vi "try_Select Enum Item.vi"() -> ()   [LabVIEW 2020]
panel:
  in  "Enum":T1(ring)
  # "Scenario\nWhen navigating an enum with a large number of items, it can be difficult to find the item you want.\n\nInstructions\n1. Right-click the enum and choose Select Item.\n2. In the UI that appears, type characters to filter the list.\n3. Select an item in the list by either double-clicking on it, or using the arrow keys and pressing Enter. The value of the enum will change to the one you selected."
  # "Close this VI when you are done with the demo."
  # "You do not need to save changes to this VI."
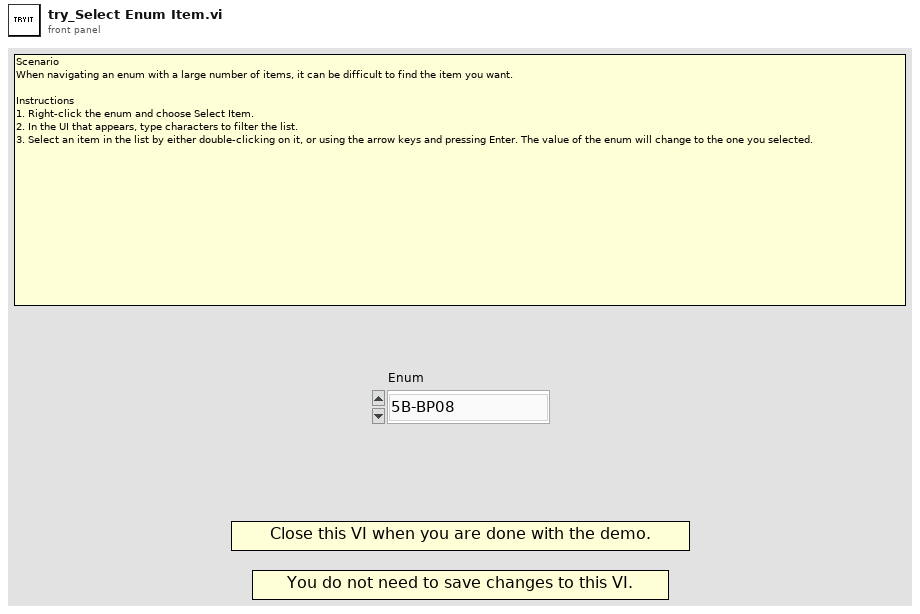
[diagram p1: front panel]
types:
  T1 = enum16{"5B-BP08", "5B-BP16", "5B30", "5B31", "5B32", "5B34", "5B37", "5B38", "5B39", "5B40", "5B41", "5B45", "5B46", "5B47", "5B49", "AMUX-64T", "AT-1120", "AT-1212", "AT-232/2", "AT-232/2 NSI", "AT-232/4", "AT-232/4 NSI", "AT-232I/2", "AT-232I/4", "AT-485/2", "AT-485/2 NSI", "AT-485/4", "AT-485/4 NSI", "AT-485I/2", "AT-485I/4", "AT-5102", "AT-5411", "AT-5431", "AT-6020/OEM1", "AT-6022E", "AT-AI-16XE-10", "AT-AO-10", "AT-AO-6", "AT-CAN", "AT-CAN/2", "AT-DIO-32F", "AT-DIO-32HS", "AT-DSP2200", "AT-GPIB", "AT-GPIB/TNT", "AT-GPIB/TNT (PnP)", "AT-GPIB/TNT+", "AT-MIO-16DE-10", "AT-MIO-16DH-25", "AT-MIO-16DH-9", "AT-MIO-16DL-25", "AT-MIO-16DL-9", "AT-MIO-16E-1", "AT-MIO-16E-10", "AT-MIO-16E-2", "AT-MIO-16F-5", "AT-MIO-16H-15", "AT-MIO-16H-25", "AT-MIO-16H-9", "AT-MIO-16L-15", "AT-MIO-16L-25", "AT-MIO-16L-9", "AT-MIO-16X", "AT-MIO-16XE-10", "AT-MIO-16XE-50", "AT-MIO-64E-3", "AT-MIO-64F-5", "AT-MXI", "AT-MXI-2", "BNC-2080", "BNC-2081", "BNC-2082", "BNC-2090", "BNC-2090A", "BNC-2095", "BNC-2096", "BNC-2110", "BNC-2111", "BNC-2115", "BNC-2120", "BNC-2121", "BNC-2140", "BNC-2142", "CAL-4353", "CB-100", "CB-27", "CB-27T", "CB-37F-HVD", "CB-50", "CB-50LC", "CB-50LP", "CB-68LP", "CB-68LPR", "CB-68T", "CEC USBDAQ/108", "CEC USBDAQ/109", "CF-6004", "CVS-1450", "CVS-1451RT", "CVS-1454", "CVS-1455", "CVS-1457RT", "CVS-1458RT", "CVS-1459RT", "CompactRIO PROFINET Slave Module", "DAQCard-1200", "DAQCard-4050", "DAQCard-4350", "DAQCard-4502", "DAQCard-500", "DAQCard-5102", "DAQCard-516", "DAQCard-5402", "DAQCard-6023E", "DAQCard-6024E", "DAQCard-6034E", "DAQCard-6035E", "DAQCard-6036E", "DAQCard-6062E", "DAQCard-6533", "DAQCard-6601", "DAQCard-6715", "DAQCard-6830", "DAQCard-700", "DAQCard-AI-16E-4", "DAQCard-AI-16XE-50", "DAQCard-AO-2DC", "DAQCard-DIO-24", "DAQPad-1200", "DAQPad-4350 for USB", "DAQPad-4351 for IEEE 1394", "DAQPad-4352 for USB", "DAQPad-5102", "DAQPad-5112 for IEEE 1394", "DAQPad-6015 for USB", "DAQPad-6015 for USB w/BNC Term", "DAQPad-6015 for USB w/Mass Term", "DAQPad-6015 for USB w/Screw Term", "DAQPad-6016 for USB w/Screw Term", "DAQPad-6020E for USB w/BNC Term", "DAQPad-6020E for USB w/Mass Term", "DAQPad-6024E for USB w/BNC Term", "DAQPad-6024E for USB w/Mass Term", "DAQPad-6025E for USB w/BNC Term", "DAQPad-6025E for USB w/Mass Term", "DAQPad-6036E for USB w/BNC Term", "DAQPad-6036E for USB w/Mass Term", "DAQPad-6052E for Ethernet w/BNC Term", "DAQPad-6052E for Ethernet w/Mass Term", "DAQPad-6052E for IEEE 1394 w/BNC Term", "DAQPad-6052E for IEEE 1394 w/Mass Term", "DAQPad-6052E for USB w/BNC Term", "DAQPad-6052E for USB w/Mass Term", "DAQPad-6070E for IEEE 1394 w/BNC Term", "DAQPad-6070E for IEEE 1394 w/Mass Term", "DAQPad-6507 for USB", "DAQPad-6508 for USB", "DAQPad-6533 for IEEE 1394", "DAQPad-6713 for IEEE 1394 w/Mass Term", "DAQPad-MIO-16XE-50", "DAQPad-TB-52", "EISA-A2000", "EISA-GPIB", "ENET-232/2", "ENET-232/4", "ENET-485/2", "ENET-485/4", "ENET-7344", "ENET-9205", "ENET-9205 DSUB", "ENET-9206", "ENET-9211", "ENET-9213", "ENET-9215", "ENET-9215 BNC", "ENET-9219", "ENET-9234", "ENET-9237", "ENET-9421", "ENET-9421 DSUB", "ENET-9472", "ENET-9472 DSUB", "ENET-9481", "ER-16", "ER-8", "FP-1000", "FP-1001", "FP-1300", "FP-1600", "FP-1601", "FP-2000", "FP-2010", "FP-2015", "FP-3000", "FP-AI-100", "FP-AI-102", "FP-AI-110", "FP-AI-111", "FP-AI-112", "FP-AIO-600", "FP-AIO-610", "FP-AO-200", "FP-AO-210", "FP-CTR-500", "FP-CTR-502", "FP-DI-300", "FP-DI-301", "FP-DI-330", "FP-DIO-550", "FP-DO-400", "FP-DO-401", "FP-DO-403", "FP-DO-410", "FP-PG-522", "FP-PWM-520", "FP-QUAD-510", "FP-RLY-420", "FP-RLY-422", "FP-RTD-122", "FP-RTD-124", "FP-SG-140", "FP-TB-1 for USB", "FP-TC-120", "FP-TC-125", "FW-7344", "GPIB-1394", "GPIB-ENET/100", "GPIB-PCII", "GPIB-PCII/IIA", "GPIB-USB", "GPIB-USB-A", "GPIB-USB-B", "GPIB-USB-HS", "GPIB-VXI/C", "IC-3120", "IC-3121", "IC-3171", "IC-3172", "IC-3173", "ISC-1780", "ISC-1780 (Color)", "ISC-1781", "ISC-1781 (Color)", "ISC-1782", "ISC-1782 (Color)", "ISC-1783", "ISC-1783 (Color)", "Lab-PC", "Lab-PC+", "Lab-PC-1200", "Lab-PC-1200AI", "MC-DIO-24", "MC-DIO-32F", "MC-MIO-16H-15", "MC-MIO-16H-25", "MC-MIO-16L-15", "MC-MIO-16L-25", "MC-MIO-16L-9", "MCC USB-488", "NB-MIO-16H-9", "NEC-AI-16E-4", "NEC-AI-16XE-50", "NEC-GPIB/TNT", "NEC-GPIB/TNT (PnP)", "NEC-MIO-16E-4", "NEC-MIO-16XE-50", "NET2280", "NI 1483", "NI 1485", "NI 1712", "NI 1722", "NI 1732", "NI 1742", "NI 1744", "NI 1752", "NI 1754", "NI 1762", "NI 1764", "NI 1772", "NI 1772C", "NI 1774", "NI 1774C", "NI 1776", "NI 1776C", "NI 1778", "NI 17XX Series Smart Camera", "NI 2810", "NI 2811", "NI 2812", "NI 2813", "NI 2814", "NI 2815", "NI 2816", "NI 2817", "NI 2833", "NI 2834", "NI 2865", "NI 4472 for IEEE 1394", "NI 5731", "NI 5732", "NI 5733", "NI 5734", "NI 5741", "NI 5742", "NI 5751", "NI 5751B", "NI 5752", "NI 5752B", "NI 5753", "NI 5753 (-01) AC", "NI 5753 (-02) DC", "NI 5761", "NI 5771", "NI 5772", "NI 5781", "NI 5782", "NI 5782 (DC)", "NI 5783", "NI 5791", "NI 5792", "NI 5793", "NI 6224 for Ethernet w/BNC Term", "NI 6224 for Ethernet w/Mass Term", "NI 6224 for Ethernet w/SCXI Term", "NI 6225 for Ethernet", "NI 6226 for Ethernet", "NI 6581", "NI 6581B", "NI 6583", "NI 6584", "NI 6585", "NI 6585B", "NI 6587", "NI 6588", "NI 6589", "NI 7451", "NI 9145", "NI 9146", "NI 9147", "NI 9148", "NI 9149", "NI 9154", "NI 9155", "NI 9157", "NI 9159", "NI 9201", "NI 9201 D-Sub", "NI 9201 cRIO", "NI 9203", "NI 9203 cRIO", "NI 9205", "NI 9205 (DSUB)", "NI 9205 D-Sub", "NI 9205 cRIO", "NI 9206", "NI 9206 cRIO", "NI 9207", "NI 9208", "NI 9209", "NI 9210", "NI 9211", "NI 9211 cRIO", "NI 9212", "NI 9213", "NI 9214", "NI 9215", "NI 9215 (BNC)", "NI 9215 BNC", "NI 9215 cRIO", "NI 9215E", "NI 9216", "NI 9217", "NI 9217 cRIO", "NI 9218", "NI 9219", "NI 9219 LEMO", "NI 9219 cRIO", "NI 9219E", "NI 9220", "NI 9220 cDAQ", "NI 9221", "NI 9221 (DSUB)", "NI 9221 (DSUB) cRIO", "NI 9221 cRIO", "NI 9222", "NI 9223", "NI 9223 cDAQ", "NI 9224", "NI 9225", "NI 9225 cRIO", "NI 9226", "NI 9227", "NI 9228", "NI 9229", "NI 9229 (BNC)", "NI 9229 BNC", "NI 9229 cRIO", "NI 9230", "NI 9230 BNC cDAQ", "NI 9232", "NI 9232 BNC cDAQ", "NI 9232 cDAQ", "NI 9232E", "NI 9233", "NI 9234", "NI 9234B", "NI 9234E", "NI 9235", "NI 9236", "NI 9237", "NI 9237 cRIO", "NI 9237 with D-Sub", "NI 9238", "NI 9239", "NI 9239 (BNC)", "NI 9239 BNC", "NI 9239 cRIO", "NI 9242", "NI 9244", "NI 9246", "NI 9247", "NI 9250", "NI 9251", "NI 9251 Mini XLR cDAQ", "NI 9260", "NI 9263", "NI 9263 (BNC)", "NI 9263 cRIO", "NI 9264", "NI 9264 D-sub", "NI 9264 cRIO", "NI 9265", "NI 9265 cRIO", "NI 9265E", "NI 9266", "NI 9269", "NI 9344", "NI 9361", "NI 9375", "NI 9375 (DSUB)", "NI 9381 DSUB", "NI 9401", "NI 9401 cRIO", "NI 9402", "NI 9402 cRIO", "NI 9403", "NI 9403 cRIO", "NI 9411", "NI 9411 cRIO", "NI 9421", "NI 9421 (DSUB)", "NI 9421 D-Sub", "NI 9421 cRIO", "NI 9422", "NI 9422 cRIO", "NI 9423", "NI 9423 cRIO", "NI 9425", "NI 9425 cRIO", "NI 9426", "NI 9426 cRIO", "NI 9435", "NI 9435 cRIO", "NI 9436", "NI 9437", "NI 9467", "NI 9469", "NI 9472", "NI 9472 (DSUB)", "NI 9472 D-Sub", "NI 9472 cRIO", "NI 9474", "NI 9474 cRIO", "NI 9475", "NI 9476", "NI 9476 cRIO", "NI 9477", "NI 9477 cRIO", "NI 9478 cRIO", "NI 9481", "NI 9481 cRIO", "NI 9481E", "NI 9482", "NI 9485", "NI 9485 cRIO", "NI 9501", "NI 9502", "NI 9503", "NI 9505", "NI 9512", "NI 9514", "NI 9516", "NI 9770", "NI 9775", "NI 9792", "NI 9795", "NI 9802 cRIO", "NI 9841", "NI 9853", "NI 9860", "NI 9861", "NI 9862", "NI 9866", "NI 9870 cRIO", "NI 9870E", "NI 9871 cRIO", "NI 9871E", "NI Bluetooth Toolkit", "NI CAN Interfaces (Series 2)", "NI CVS-1450 Series", "NI DeviceNet Interfaces", "NI ELVIS II", "NI ELVIS II+", "NI EVS-1460 Series", "NI ExpressCard-8360", "NI ExpressCard-8420/2", "NI ExpressCard-8421/2", "NI ExpressCard-GPIB", "NI PCI-8511 CAN/LS1", "NI PCI-8511 CAN/LS2", "NI PCI-8512 CAN/HS1", "NI PCI-8512 CAN/HS2", "NI PCI-8513 CAN/XS1", "NI PCI-8513 CAN/XS2", "NI PCI-8516 LIN/2", "NI PCI-8517 FlexRay2", "NI PCIe-1427", "NI PCIe-1429", "NI PCIe-1430", "NI PCIe-1433", "NI PCIe-4065", "NI PCIe-5122", "NI PCIe-5142", "NI PCIe-6250", "NI PCIe-6251", "NI PCIe-6259", "NI PCIe-6344R", "NI PCIe-6346R", "NI PCIe-6509", "NI PCIe-6535", "NI PCIe-6536", "NI PCIe-6537", "NI PCIe-6542", "NI PCIe-6552", "NI PCIe-8231", "NI PCIe-8235", "NI PCIe-8253", "NI PCIe-8255R", "NI PCIe-GPIB", "NI PXI-4110", "NI PXI-4130", "NI PXI-4131A", "NI PXI-4132", "NI PXI-8511 CAN/LS1", "NI PXI-8511 CAN/LS2", "NI PXI-8512 CAN/HS1", "NI PXI-8512 CAN/HS2", "NI PXI-8513 CAN/XS1", "NI PXI-8513 CAN/XS2", "NI PXI-8516 LIN/2", "NI PXI-8517 FlexRay2", "NI PXIe-1062Q", "NI PXIe-1065", "NI PXIe-1436", "NI PXIe-1491", "NI PXIe-4112", "NI PXIe-4113", "NI PXIe-4136", "NI PXIe-4137", "NI PXIe-4138", "NI PXIe-4139", "NI PXIe-4140", "NI PXIe-4141", "NI PXIe-4142", "NI PXIe-4143", "NI PXIe-4144", "NI PXIe-4145", "NI PXIe-4154", "NI PXIe-4496", "NI PXIe-4498", "NI PXIe-5122", "NI PXIe-5142", "NI PXIe-5421", "NI PXIe-5422", "NI PXIe-5442", "NI PXIe-5450", "NI PXIe-5451", "NI PXIe-5452", "NI PXIe-5453", "NI PXIe-5455", "NI PXIe-5602", "NI PXIe-5612", "NI PXIe-5622", "NI PXIe-6251", "NI PXIe-6259", "NI PXIe-6535", "NI PXIe-6536", "NI PXIe-6537", "NI PXIe-6542", "NI PXIe-6552", "NI PXIe-8103", "NI PXIe-8105", "NI PXIe-8106", "NI PXIe-8130", "NI PXIe-8131", "NI PXIe-8234", "NI SoftMotion Controller for CANopen", "NI SoftMotion Controller for IEEE 1394", "NI TBX-2808", "NI USB 7845R", "NI USB 7845R OEM", "NI USB 7846R OEM", "NI USB-6341", "NI USB-6341 OEM", "NI USB-6343", "NI USB-6343 OEM", "NI USB-6351", "NI USB-6353", "NI USB-6356 (32 MS) (Screw Terminal)", "NI USB-6356 (32MS)", "NI USB-6356 (32MS) OEM", "NI USB-6356 (64 MS) (Screw Terminal)", "NI USB-6356 (64MS)", "NI USB-6361", "NI USB-6361 OEM", "NI USB-6363", "NI USB-6363 OEM", "NI USB-6366 (32 MS) (Screw Terminal)", "NI USB-6366 (32MS)", "NI USB-6366 (64 MS) (Screw Terminal)", "NI USB-6366 (64MS)", "NI USB-6366 (64MS) OEM", "NI USB-7846R", "NI USB-7855R", "NI USB-7855R OEM", "NI USB-7856R", "NI USB-7856R OEM", "NI USB-TC01", "NI USRP-2944R", "NI USRP-2954R", "NI WSN-3202", "NI WSN-3202 (programmable)", "NI WSN-3212", "NI WSN-3212 (programmable)", "NI WSN-3214", "NI WSN-3214 LV", "NI WSN-3226", "NI WSN-3226 (programmable)", "NI WSN-3230", "NI WSN-3231", "NI WSN-3234", "NI WSN-3234 LV", "NI WSN-9791", "NI WSN-9792 OEM", "NI myDAQ", "NI myDAQ Hardware", "NI myRIO", "NI roboRIO", "NI-1702", "NI-7931", "NI-7932", "NI-7935", "NI-9852", "NI-IMAQ for IEEE 1394 Cameras", "OEM USB-7931R", "OEM USB-7932R", "OEM USB-7933R", "PC-4350", "PC-516", "PC-AO-2DC", "PC-DIO-24", "PC-DIO-96", "PC-DIO-96PnP", "PC-FlexMotion-6C", "PC-LPM-16", "PC-LPM-16PnP", "PC-OPDIO-16", "PC-Servo-1P", "PC-Servo-2A", "PC-Servo-4A", "PC-Step-2CX", "PC-Step-2OX", "PC-Step-4CX", "PC-Step-4OX", "PC-TIO-10", "PCI-1200", "PCI-1405", "PCI-1407", "PCI-1408", "PCI-1409", "PCI-1410", "PCI-1411", "PCI-1412", "PCI-1413", "PCI-1422", "PCI-1423", "PCI-1424", "PCI-1426", "PCI-1428", "PCI-1588", "PCI-232/16", "PCI-232/2", "PCI-232/4", "PCI-232/8", "PCI-232I/2", "PCI-232I/4", "PCI-4021", "PCI-4060", "PCI-4065", "PCI-4070", "PCI-4351", "PCI-4451", "PCI-4452", "PCI-4453", "PCI-4454", "PCI-4461", "PCI-4462", "PCI-4472", "PCI-4472B", "PCI-4474", "PCI-4551", "PCI-4552", "PCI-485/2", "PCI-485/4", "PCI-485/8", "PCI-485I/2", "PCI-485I/4", "PCI-488", "PCI-488LP", "PCI-5102", "PCI-5104", "PCI-5105", "PCI-5112", "PCI-5114", "PCI-5122", "PCI-5124", "PCI-5142", "PCI-5152", "PCI-5153", "PCI-5154", "PCI-5401", "PCI-5402", "PCI-5406", "PCI-5411", "PCI-5412", "PCI-5420", "PCI-5421", "PCI-5422", "PCI-5431", "PCI-5640R", "PCI-5911", "PCI-5922", "PCI-5922EX", "PCI-6010", "PCI-6011E", "PCI-6013", "PCI-6014", "PCI-6023E", "PCI-6024E", "PCI-6025E", "PCI-6030E", "PCI-6031E", "PCI-6032E", "PCI-6033E", "PCI-6034E", "PCI-6035E", "PCI-6036E", "PCI-6040E (PCI-MIO-16E-4)", "PCI-6052E", "PCI-6053E", "PCI-6070E", "PCI-6071E", "PCI-6110", "PCI-6111", "PCI-6115", "PCI-6120", "PCI-6122", "PCI-6123", "PCI-6132", "PCI-6133", "PCI-6143", "PCI-6154", "PCI-6220", "PCI-6221", "PCI-6221 (37-Pin)", "PCI-6222", "PCI-6224", "PCI-6225", "PCI-6229", "PCI-6230", "PCI-6232", "PCI-6233", "PCI-6236", "PCI-6238", "PCI-6239", "PCI-6250", "PCI-6251", "PCI-6254", "PCI-6255", "PCI-6259", "PCI-6280", "PCI-6281", "PCI-6284", "PCI-6289", "PCI-6503", "PCI-6504", "PCI-6505", "PCI-6509", "PCI-6510", "PCI-6511", "PCI-6512", "PCI-6513", "PCI-6514", "PCI-6515", "PCI-6516", "PCI-6517", "PCI-6518", "PCI-6519", "PCI-6520", "PCI-6521", "PCI-6525", "PCI-6526", "PCI-6527", "PCI-6528", "PCI-6533", "PCI-6534", "PCI-6541", "PCI-6542", "PCI-6551", "PCI-6552", "PCI-6561", "PCI-6562", "PCI-6601", "PCI-6602", "PCI-6608", "PCI-6610", "PCI-6624", "PCI-6703", "PCI-6704", "PCI-6711", "PCI-6713", "PCI-6722", "PCI-6723", "PCI-6731", "PCI-6733", "PCI-6810", "PCI-7030/6030E", "PCI-7030/6040E", "PCI-7040/6040E", "PCI-7041/6040E", "PCI-716", "PCI-7314", "PCI-7324", "PCI-7330", "PCI-7332", "PCI-7334", "PCI-7340", "PCI-7342", "PCI-7344", "PCI-7346", "PCI-7350", "PCI-7390", "PCI-7414", "PCI-7811R", "PCI-7813R", "PCI-7830R", "PCI-7831R", "PCI-7833R", "PCI-7841R", "PCI-7842R", "PCI-7851R", "PCI-7852R", "PCI-7853R", "PCI-8215", "PCI-8252", "PCI-8254R", "PCI-8320", "PCI-8410/2", "PCI-8430/16", "PCI-8430/2", "PCI-8430/4", "PCI-8430/8", "PCI-8431/2", "PCI-8431/4", "PCI-8431/8", "PCI-8432/2", "PCI-8432/4", "PCI-8433/2", "PCI-8433/4", "PCI-CAN", "PCI-CAN (DNET)", "PCI-CAN Series 2", "PCI-CAN/2", "PCI-CAN/2 Series 2", "PCI-CAN/DS", "PCI-CAN/DS Series 2", "PCI-CAN/LS", "PCI-CAN/LS Series 2", "PCI-CAN/LS2", "PCI-CAN/LS2 Series 2", "PCI-CAN/SW Series 2", "PCI-CAN/SW2 Series 2", "PCI-CAN/XS Series 2", "PCI-CAN/XS2 Series 2", "PCI-DIO-32HS-T", "PCI-DIO-96", "PCI-FBUS", "PCI-FBUS/2", "PCI-FlexMotion-6C", "PCI-GPIB", "PCI-GPIB+", "PCI-MXI-2", "PCI-MXI-2 Universal", "PCI-Servo-2A", "PCI-Servo-4A", "PCI-Step-2CX", "PCI-Step-2OX", "PCI-Step-4CX", "PCI-Step-4OX", "PCIe-1433R", "PCIe-1434R", "PCIe-1435R", "PCIe-1436R", "PCIe-1473R", "PCIe-1473R-LX110", "PCIe-1474R", "PCIe-1475R", "PCIe-1476R", "PCIe-6320", "PCIe-6321", "PCIe-6323", "PCIe-6326", "PCIe-6341", "PCIe-6343", "PCIe-6346", "PCIe-6351", "PCIe-6353", "PCIe-6356", "PCIe-6361", "PCIe-6363", "PCIe-6612", "PCIe-8233", "PCIe-8236", "PCIe-8237R", "PCIe-8242", "PCIe-8244", "PCIe-8430/16", "PCIe-8430/8", "PCIe-8431/16", "PCIe-8431/8", "PCIe-GPIB+", "PCMCIA-232", "PCMCIA-232 921.6k", "PCMCIA-232/2", "PCMCIA-232/2 921.6k", "PCMCIA-232/4", "PCMCIA-485", "PCMCIA-485 921.6k", "PCMCIA-485/2", "PCMCIA-485/2 921.6k", "PCMCIA-6024E", "PCMCIA-6036E", "PCMCIA-6062E", "PCMCIA-CAN", "PCMCIA-CAN (DNET)", "PCMCIA-CAN Series 2", "PCMCIA-CAN/2", "PCMCIA-CAN/2 Series 2", "PCMCIA-CAN/LS", "PCMCIA-CAN/LS2", "PCMCIA-FBUS", "PCMCIA-FBUS Series 2", "PCMCIA-FBUS/2", "PCMCIA-FBUS/2 Series 2", "PCMCIA-GPIB", "PCMCIA-GPIB+", "PMC-GPIB", "PSH32-TC6", "PXI-1010", "PXI-1011", "PXI-1033", "PXI-1044", "PXI-1045", "PXI-1050", "PXI-1052", "PXI-1056", "PXI-1405", "PXI-1407", "PXI-1408", "PXI-1409", "PXI-1411", "PXI-1412", "PXI-1413", "PXI-1422", "PXI-1423", "PXI-1424", "PXI-1428", "PXI-1588", "PXI-2501", "PXI-2503", "PXI-2510", "PXI-2512", "PXI-2514", "PXI-2515", "PXI-2520", "PXI-2521", "PXI-2522", "PXI-2523", "PXI-2527", "PXI-2528", "PXI-2529", "PXI-2530", "PXI-2531", "PXI-2532", "PXI-2533", "PXI-2534", "PXI-2535", "PXI-2536", "PXI-2537", "PXI-2538", "PXI-2540", "PXI-2541", "PXI-2542", "PXI-2543", "PXI-2544", "PXI-2545", "PXI-2546", "PXI-2547", "PXI-2548", "PXI-2549", "PXI-2554", "PXI-2555", "PXI-2556", "PXI-2557", "PXI-2558", "PXI-2559", "PXI-2564", "PXI-2565", "PXI-2566", "PXI-2567", "PXI-2568", "PXI-2569", "PXI-2570", "PXI-2571", "PXI-2575", "PXI-2576", "PXI-2584", "PXI-2585", "PXI-2586", "PXI-2590", "PXI-2591", "PXI-2593", "PXI-2594", "PXI-2595", "PXI-2596", "PXI-2597", "PXI-2598", "PXI-2599", "PXI-2720", "PXI-2722", "PXI-2796", "PXI-2797", "PXI-2798", "PXI-2799", "PXI-2810", "PXI-2811", "PXI-2812", "PXI-2813", "PXI-2814", "PXI-2815", "PXI-2816", "PXI-2817", "PXI-2833", "PXI-2834", "PXI-2865", "PXI-4021", "PXI-4022", "PXI-4060", "PXI-4065", "PXI-4070", "PXI-4071", "PXI-4072", "PXI-4130SL", "PXI-4170", "PXI-4200", "PXI-4204", "PXI-4220", "PXI-4224", "PXI-4225", "PXI-4351", "PXI-4411", "PXI-4461", "PXI-4461 eHM", "PXI-4462", "PXI-4462 eHM", "PXI-4472", "PXI-4472B", "PXI-4474", "PXI-4492", "PXI-4494", "PXI-4495", "PXI-4496", "PXI-4498", "PXI-4551", "PXI-4552", "PXI-485/8", "PXI-5102", "PXI-5104", "PXI-5105", "PXI-5112", "PXI-5114", "PXI-5122", "PXI-5124", "PXI-5142", "PXI-5152", "PXI-5153", "PXI-5154", "PXI-5401", "PXI-5402", "PXI-5404", "PXI-5406", "PXI-5411", "PXI-5412", "PXI-5420", "PXI-5421", "PXI-5422", "PXI-5431", "PXI-5433", "PXI-5441", "PXI-5600", "PXI-5610", "PXI-5620", "PXI-5621", "PXI-5650", "PXI-5651", "PXI-5652", "PXI-5653", "PXI-5660", "PXI-5661", "PXI-5670", "PXI-5671", "PXI-5690", "PXI-5691", "PXI-5695", "PXI-5900", "PXI-5911", "PXI-5922", "PXI-5922EX", "PXI-6011E", "PXI-6023E", "PXI-6024E", "PXI-6025E", "PXI-6030E", "PXI-6031E", "PXI-6032E", "PXI-6033E", "PXI-6035E", "PXI-6040E", "PXI-6052E", "PXI-6053E", "PXI-6070E", "PXI-6071E", "PXI-6115", "PXI-6120", "PXI-6122", "PXI-6123", "PXI-6132", "PXI-6133", "PXI-6143", "PXI-6220", "PXI-6221", "PXI-6222", "PXI-6224", "PXI-6225", "PXI-6229", "PXI-6230", "PXI-6232", "PXI-6233", "PXI-6236", "PXI-6238", "PXI-6239", "PXI-6250", "PXI-6251", "PXI-6254", "PXI-6255", "PXI-6259", "PXI-6280", "PXI-6281", "PXI-6284", "PXI-6289", "PXI-6503", "PXI-6504", "PXI-6505", "PXI-6508", "PXI-6509", "PXI-6511", "PXI-6512", "PXI-6513", "PXI-6514", "PXI-6515", "PXI-6521", "PXI-6525", "PXI-6526", "PXI-6527", "PXI-6528", "PXI-6529", "PXI-6533", "PXI-6534", "PXI-6541", "PXI-6542", "PXI-6551", "PXI-6552", "PXI-6561", "PXI-6562", "PXI-6601", "PXI-6602", "PXI-6608", "PXI-6610", "PXI-6624", "PXI-6651", "PXI-6652", "PXI-6653", "PXI-6682", "PXI-6682H", "PXI-6683", "PXI-6683H", "PXI-6684", "PXI-6684H", "PXI-6685", "PXI-6685H", "PXI-6703", "PXI-6704", "PXI-6711", "PXI-6713", "PXI-6722", "PXI-6723", "PXI-6731", "PXI-6733", "PXI-6810", "PXI-6830", "PXI-7030/6030E", "PXI-7040/6040E", "PXI-7041/6040E", "PXI-7312", "PXI-7314", "PXI-7322", "PXI-7324", "PXI-7330", "PXI-7332", "PXI-7334", "PXI-7340", "PXI-7342", "PXI-7344", "PXI-7346", "PXI-7350", "PXI-7811R", "PXI-7813R", "PXI-7830R", "PXI-7831R", "PXI-7833R", "PXI-7841R", "PXI-7842R", "PXI-7851R", "PXI-7852R", "PXI-7853R", "PXI-7854R", "PXI-7951R", "PXI-7952R", "PXI-7953R", "PXI-7954R", "PXI-8105", "PXI-8106", "PXI-8107", "PXI-8108", "PXI-8110", "PXI-8115", "PXI-8119", "PXI-8156B", "PXI-8184", "PXI-8195", "PXI-8250", "PXI-8252", "PXI-8320", "PXI-8352", "PXI-8420/16", "PXI-8420/2", "PXI-8420/4", "PXI-8420/8", "PXI-8421/2", "PXI-8421/4", "PXI-8422/2", "PXI-8422/4", "PXI-8423/2", "PXI-8423/4", "PXI-8430/16", "PXI-8430/2", "PXI-8430/4", "PXI-8430/8", "PXI-8431/2", "PXI-8431/4", "PXI-8431/8", "PXI-8432/2", "PXI-8432/4", "PXI-8433/2", "PXI-8433/4", "PXI-8460/1", "PXI-8460/1 Series 2", "PXI-8460/2", "PXI-8460/2 Series 2", "PXI-8461 (DNET)", "PXI-8461/1", "PXI-8461/1 Series 2", "PXI-8461/2", "PXI-8461/2 Series 2", "PXI-8462", "PXI-8462 Series 2", "PXI-8463/1 Series 2", "PXI-8463/2 Series 2", "PXI-8464/1", "PXI-8464/2 Series 2", "PXI-8533", "PXI-GPIB", "PXIe-1435", "PXIe-2512", "PXIe-2514", "PXIe-2515", "PXIe-2524", "PXIe-2525", "PXIe-2526", "PXIe-2527", "PXIe-2529", "PXIe-2530", "PXIe-2531", "PXIe-2532", "PXIe-2540", "PXIe-2541", "PXIe-2542", "PXIe-2543", "PXIe-2544", "PXIe-2569", "PXIe-2575", "PXIe-2593", "PXIe-2725", "PXIe-2727", "PXIe-2737", "PXIe-2738", "PXIe-2739", "PXIe-2746", "PXIe-2747", "PXIe-2748", "PXIe-2790", "PXIe-3610", "PXIe-3620", "PXIe-3630", "PXIe-3647", "PXIe-3657", "PXIe-4080", "PXIe-4081", "PXIe-4082", "PXIe-4135", "PXIe-4300", "PXIe-4302", "PXIe-4303", "PXIe-4304", "PXIe-4305", "PXIe-4309", "PXIe-4310", "PXIe-4322", "PXIe-4330", "PXIe-4331", "PXIe-4339", "PXIe-4340", "PXIe-4353", "PXIe-4357", "PXIe-4463", "PXIe-4464", "PXIe-4480", "PXIe-4481", "PXIe-4492", "PXIe-4497", "PXIe-4499", "PXIe-4844 (OSI)", "PXIe-5105", "PXIe-5114", "PXIe-5160 (2 ch)", "PXIe-5160 (4 ch)", "PXIe-5162 (2 ch)", "PXIe-5162 (4 ch)", "PXIe-5164", "PXIe-5170R", "PXIe-5171R", "PXIe-5172", "PXIe-5185 (1 MOhm)", "PXIe-5185 (50 Ohm)", "PXIe-5186 (1 MOhm)", "PXIe-5186 (50 Ohm)", "PXIe-5601", "PXIe-5603", "PXIe-5605", "PXIe-5606", "PXIe-5611", "PXIe-5624", "PXIe-5630", "PXIe-5632", "PXIe-5641R", "PXIe-5644R", "PXIe-5645R", "PXIe-5646R", "PXIe-5650", "PXIe-5651", "PXIe-5652", "PXIe-5653", "PXIe-5654", "PXIe-5663", "PXIe-5663E", "PXIe-5665 14GHz", "PXIe-5665 3.6GHz", "PXIe-5667 3.6GHz", "PXIe-5667 7GHz", "PXIe-5668R", "PXIe-5672", "PXIe-5673", "PXIe-5693", "PXIe-5694", "PXIe-5698", "PXIe-5840", "PXIe-6124", "PXIe-6341", "PXIe-6346", "PXIe-6356", "PXIe-6358", "PXIe-6361", "PXIe-6363", "PXIe-6366", "PXIe-6368", "PXIe-6376", "PXIe-6378", "PXIe-6544", "PXIe-6545", "PXIe-6547", "PXIe-6548", "PXIe-6555", "PXIe-6556", "PXIe-6570", "PXIe-6612", "PXIe-6614", "PXIe-6672", "PXIe-6674", "PXIe-6674T", "PXIe-6738", "PXIe-6739", "PXIe-7820R", "PXIe-7821R", "PXIe-7822R", "PXIe-7846R", "PXIe-7847R", "PXIe-7856R", "PXIe-7857R", "PXIe-7858R", "PXIe-7961R", "PXIe-7962R", "PXIe-7965R", "PXIe-7966R", "PXIe-7971R", "PXIe-7972R", "PXIe-7975R", "PXIe-7976R", "PXIe-8100", "PXIe-8115", "PXIe-8135", "PXIe-8364 (NT)", "PXIe-8374 (NT)", "PXIe-8378", "PXIe-8379", "PXIe-8383mc", "PXIe-8384", "PXIe-8388", "PXIe-8389", "PXIe-8510", "SB-A2200", "SB-MIO-16E-4", "SC-2040", "SC-2042-RTD", "SC-2043-SG", "SC-2050", "SC-2051", "SC-2052", "SC-2053", "SC-2054", "SC-2055", "SC-2056", "SC-2060", "SC-2061", "SC-2062", "SC-2070", "SC-2071", "SC-2072", "SC-2072D", "SC-2075", "SC-2311", "SC-2345", "SC-2350", "SCB-100", "SCB-68", "SCB-68A", "SCC-68", "SCC-A10", "SCC-AI00", "SCC-AI01", "SCC-AI02", "SCC-AI03", "SCC-AI04", "SCC-AI05", "SCC-AI06", "SCC-AI07", "SCC-AI13", "SCC-AI14", "SCC-AI16", "SCC-AO10", "SCC-CI20", "SCC-CO20", "SCC-CTR01", "SCC-DI01", "SCC-DO01", "SCC-FT01", "SCC-FV01", "SCC-LP01", "SCC-LP02", "SCC-LP03", "SCC-LP04", "SCC-LP05", "SCC-PWR01", "SCC-PWR02", "SCC-PWR03", "SCC-RLY01", "SCC-RTD01", "SCC-SG01", "SCC-SG02", "SCC-SG03", "SCC-SG04", "SCC-SG11", "SCC-SG24", "SCC-TC01", "SCC-TC02", "SCC-TC03", "SCC-TC12", "SCC-TC13", "SCMP-100uA", "SCMP-10V", "SCMP-10uA", "SCMP-13mA", "SCMP-1V", "SCMP-1mA", "SCMP-2V", "SCMP-5V", "SCXI-1000", "SCXI-1000DC", "SCXI-1001", "SCXI-1100", "SCXI-1101", "SCXI-1102", "SCXI-1102B", "SCXI-1102C", "SCXI-1104", "SCXI-1104C", "SCXI-1112", "SCXI-1120", "SCXI-1120D", "SCXI-1121", "SCXI-1122", "SCXI-1124", "SCXI-1125", "SCXI-1126", "SCXI-1127", "SCXI-1128", "SCXI-1129", "SCXI-1130", "SCXI-1140", "SCXI-1141", "SCXI-1142", "SCXI-1143", "SCXI-1160", "SCXI-1160A", "SCXI-1161", "SCXI-1162", "SCXI-1162HV", "SCXI-1163", "SCXI-1163R", "SCXI-1166", "SCXI-1167", "SCXI-1169", "SCXI-1175", "SCXI-1190", "SCXI-1191", "SCXI-1192", "SCXI-1193", "SCXI-1194", "SCXI-1195", "SCXI-1200", "SCXI-1300", "SCXI-1301", "SCXI-1302", "SCXI-1303", "SCXI-1304", "SCXI-1305", "SCXI-1306", "SCXI-1307", "SCXI-1308", "SCXI-1310", "SCXI-1311", "SCXI-1313", "SCXI-1314", "SCXI-1314T", "SCXI-1315", "SCXI-1317", "SCXI-1320", "SCXI-1321", "SCXI-1322", "SCXI-1323", "SCXI-1324", "SCXI-1325", "SCXI-1326", "SCXI-1327", "SCXI-1328", "SCXI-1330", "SCXI-1331", "SCXI-1332", "SCXI-1333", "SCXI-1334", "SCXI-1335", "SCXI-1336", "SCXI-1337", "SCXI-1338", "SCXI-1339", "SCXI-1357", "SCXI-1366", "SCXI-1377", "SCXI-1378", "SCXI-1379", "SCXI-1502", "SCXI-1503", "SCXI-1520", "SCXI-1521", "SCXI-1521B", "SCXI-1530", "SCXI-1531", "SCXI-1540", "SCXI-1581", "SCXI-1600", "SCXI-2000", "SCXI-2400", "SSR-BP16", "SSR-BP24", "SSR-BP32", "SSR-BP8", "SSR-IAC-5", "SSR-IAC-5A", "SSR-IDC-5", "SSR-OAC-5", "SSR-OAC-5A", "SSR-ODC-5", "SensorDAQ", "TB-2130", "TB-2605", "TB-2606", "TB-2621", "TB-2627", "TB-2630", "TB-2630B", "TB-2631", "TB-2632", "TB-2634", "TB-2635", "TB-2636", "TB-2640", "TB-2641", "TB-2642", "TB-2643", "TB-2644", "TB-2645", "TB-2646", "TB-2666", "TB-2676", "TB-2705", "TB-2706", "TB-2708", "TB-2709", "TB-2715", "TB-2725", "TB-4300C", "TB-4302", "TB-4302C", "TB-4304", "TB-4339", "TB-4339B", "TB-4339C", "TB-4357", "TBX-1303", "TBX-1316", "TBX-1325", "TBX-1326", "TBX-1328", "TBX-1329", "TBX-2131", "TBX-24F", "TBX-68", "TBX-68T", "TBX-96", "TC-2095", "TC-2190", "TC-4353", "USB-1359", "USB-232", "USB-232/2", "USB-232/4", "USB-4065", "USB-4431", "USB-4432", "USB-4444", "USB-485", "USB-485/2", "USB-485/4", "USB-488", "USB-5132", "USB-5133", "USB-5134", "USB-5680", "USB-5681", "USB-5683", "USB-5684", "USB-6000", "USB-6000 OEM", "USB-6002", "USB-6002 OEM", "USB-6003", "USB-6003 OEM", "USB-6005", "USB-6005 OEM", "USB-6005 VSA", "USB-6008", "USB-6009", "USB-6009 OEM", "USB-6210", "USB-6210 OEM", "USB-6211", "USB-6211 OEM", "USB-6212", "USB-6212 BNC", "USB-6212 Mass Term", "USB-6212 OEM", "USB-6215", "USB-6215 OEM", "USB-6216", "USB-6216 BNC", "USB-6216 Mass Term", "USB-6216 OEM", "USB-6218", "USB-6218 BNC", "USB-6218 OEM", "USB-6220", "USB-6220 Mass Term", "USB-6220 OEM", "USB-6221", "USB-6221 (BNC)", "USB-6221 BNC", "USB-6221 Mass Term", "USB-6221 OEM", "USB-6224", "USB-6224 Mass Term", "USB-6224 OEM", "USB-6225", "USB-6225 Mass Term", "USB-6229", "USB-6229 (BNC)", "USB-6229 BNC", "USB-6229 Mass Term", "USB-6229 OEM", "USB-6250", "USB-6250 Mass Term", "USB-6250 OEM", "USB-6251", "USB-6251 (BNC)", "USB-6251 BNC", "USB-6251 Mass Term", "USB-6251 OEM", "USB-6254", "USB-6254 Mass Term", "USB-6254 OEM", "USB-6255", "USB-6255 Mass Term", "USB-6259", "USB-6259 (BNC)", "USB-6259 BNC", "USB-6259 Mass Term", "USB-6259 OEM", "USB-6281", "USB-6281 (Mass Termination)", "USB-6281 BNC", "USB-6281 Mass Term", "USB-6289", "USB-6289 (Mass Termination)", "USB-6289 BNC", "USB-6289 Mass Term", "USB-6326", "USB-6341 BNC", "USB-6343 BNC", "USB-6343 OEM RTSI", "USB-6346", "USB-6356 (32MS) BNC", "USB-6356 (32MS) OEM RTSI", "USB-6361 BNC", "USB-6363 BNC", "USB-6363 Mass Term RTSI", "USB-6366 (64MS) BNC", "USB-6501", "USB-6504", "USB-6509", "USB-6525", "USB-7931R", "USB-7932R", "USB-7933R", "USB-8451", "USB-8452", "USB-8472", "USB-8472s", "USB-8473", "USB-8473s", "USB-8476", "USB-8476s", "USB-8502", "USB-8506", "USB-9161", "USB-9162", "USB-9201", "USB-9201 D-Sub", "USB-9211", "USB-9211A", "USB-9213", "USB-9215", "USB-9215A", "USB-9215A BNC", "USB-9221", "USB-9229 (BNC)", "USB-9233", "USB-9234", "USB-9237", "USB-9239 (BNC)", "USB-9263 (BNC)", "USB-9264 D-SUB", "USB-9421", "USB-9421 D-Sub", "USB-9421DSUB", "USB-9472", "USB-9472 D-Sub", "USB-9472DSUB", "USB-9481", "VMEpc-650", "VXI-1394", "VXI-2701", "VXI-2703", "VXI-2727", "VXI-5412", "VXI-5432", "VXI-5912", "VXI-8340", "VXI-8345", "VXI-AO-48XDC", "VXI-DIO-128", "VXI-MIO-64E-1", "VXI-MIO-64XE-10", "VXI-SC-1000", "VXI-SC-1102", "VXI-SC-1102B", "VXI-SC-1102C", "VXI-SC-1150", "VXI-TB-1303", "VXI-TB-96", "VXI-USB", "VXIpc-650", "VXIpc-740", "VXIpc-770", "VXIpc-850", "VXIpc-860", "VXIpc-870", "VXIpc-870B", "VXIpc-881", "WLAN Toolkit", "WLS-9205", "WLS-9205 DSUB", "WLS-9206", "WLS-9211", "WLS-9213", "WLS-9215", "WLS-9215 BNC", "WLS-9219", "WLS-9234", "WLS-9237", "WLS-9421", "WLS-9421 DSUB", "WLS-9472", "WLS-9472 DSUB", "WLS-9481", "cDAQ-9171", "cDAQ-9171 OEM", "cDAQ-9172", "cDAQ-9174", "cDAQ-9178", "cDAQ-9181", "cDAQ-9184", "cDAQ-9188", "cDAQ-9191", "cFP-1804", "cFP-1808", "cFP-2000", "cFP-2010", "cFP-2020", "cFP-2100", "cFP-2110", "cFP-2120", "cFP-2200", "cFP-AI-100", "cFP-AI-102", "cFP-AI-110", "cFP-AI-111", "cFP-AI-112", "cFP-AI-118", "cFP-AIO-600", "cFP-AIO-610", "cFP-AO-200", "cFP-AO-210", "cFP-CTR-500", "cFP-CTR-502", "cFP-DI-300", "cFP-DI-301", "cFP-DI-304", "cFP-DI-330", "cFP-DIO-550", "cFP-DO-400", "cFP-DO-401", "cFP-DO-403", "cFP-DO-404", "cFP-DO-410", "cFP-PG-522", "cFP-PWM-520", "cFP-QUAD-510", "cFP-RLY-420", "cFP-RLY-421", "cFP-RLY-422", "cFP-RLY-423", "cFP-RLY-425", "cFP-RTD-122", "cFP-RTD-124", "cFP-SG-140", "cFP-TC-120", "cFP-TC-125", "cRIO-9002", "cRIO-9004", "cRIO-9012", "cRIO-9014", "cRIO-9022", "cRIO-9023", "cRIO-9024", "cRIO-9025", "cRIO-9030", "cRIO-9031", "cRIO-9032", "cRIO-9033", "cRIO-9034", "cRIO-9035", "cRIO-9036", "cRIO-9037", "cRIO-9038", "cRIO-9039", "cRIO-9063", "cRIO-9064", "cRIO-9065", "cRIO-9066", "cRIO-9067", "cRIO-9068", "cRIO-9072", "cRIO-9073", "cRIO-9074", "cRIO-9075", "cRIO-9076", "cRIO-9077", "cRIO-9081", "cRIO-9082", "cRIO-9101", "cRIO-9102", "cRIO-9103", "cRIO-9104", "cRIO-9111", "cRIO-9112", "cRIO-9113", "cRIO-9114", "cRIO-9116", "cRIO-9118", "cRIO-9413", "cRIO-FRC II", "sbRIO-9601", "sbRIO-9602", "sbRIO-9603", "sbRIO-9605", "sbRIO-9606", "sbRIO-9607", "sbRIO-9611", "sbRIO-9612", "sbRIO-9623", "sbRIO-9625", "sbRIO-9626", "sbRIO-9627", "sbRIO-9631", "sbRIO-9632", "sbRIO-9633", "sbRIO-9636", "sbRIO-9637", "sbRIO-9641", "sbRIO-9642", "sbRIO-9651"}
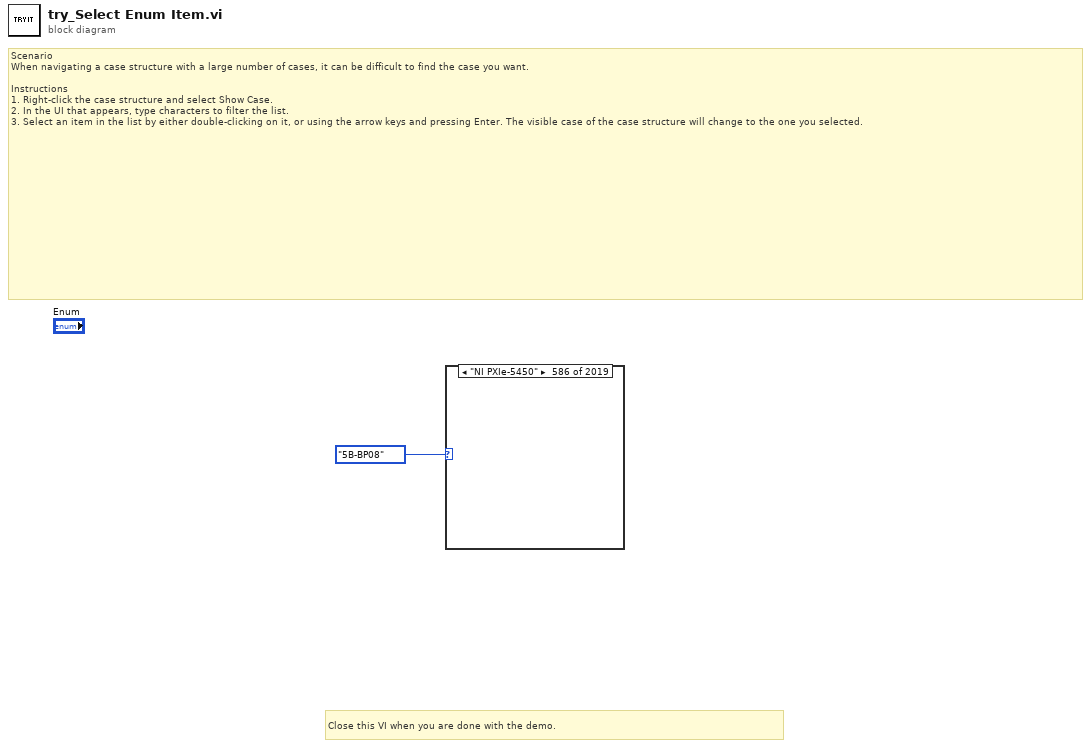
[diagram p0: block diagram]
diagram:
  # "Close this VI when you are done with the demo."
  # "Scenario\nWhen navigating a case structure with a large number of cases, it can be difficult to find the case you want.\n\nInstructions\n1. Right-click the case structure and select Show Case.\n2. In the UI that appears, type characters to filter the list.\n3. Select an item in the list by either double-clicking on it, or using the arrow keys and pressing Enter. The visible case of the case structure will change to the one you selected."
  n1 = case shown="\"NI PXIe-5450\"" T1."5B-BP08" ("Enum") {
    frame "5B-BP08", Default {
    }
    frame "5B-BP16" {
    }
    frame "5B30" {
    }
    frame "5B31" {
    }
    frame "5B32" {
    }
    frame "5B34" {
    }
    frame "5B37" {
    }
    frame "5B38" {
    }
    frame "5B39" {
    }
    frame "5B40" {
    }
    frame "5B41" {
    }
    frame "5B45" {
    }
    frame "5B46" {
    }
    frame "5B47" {
    }
    frame "5B49" {
    }
    frame "AMUX-64T" {
    }
    frame "AT-1120" {
    }
    frame "AT-1212" {
    }
    frame "AT-232/2" {
    }
    frame "AT-232/2 NSI" {
    }
    frame "AT-232/4" {
    }
    frame "AT-232/4 NSI" {
    }
    frame "AT-232I/2" {
    }
    frame "AT-232I/4" {
    }
    frame "AT-485/2" {
    }
    frame "AT-485/2 NSI" {
    }
    frame "AT-485/4" {
    }
    frame "AT-485/4 NSI" {
    }
    frame "AT-485I/2" {
    }
    frame "AT-485I/4" {
    }
    frame "AT-5102" {
    }
    frame "AT-5411" {
    }
    frame "AT-5431" {
    }
    frame "AT-6020/OEM1" {
    }
    frame "AT-6022E" {
    }
    frame "AT-AI-16XE-10" {
    }
    frame "AT-AO-10" {
    }
    frame "AT-AO-6" {
    }
    frame "AT-CAN" {
    }
    frame "AT-CAN/2" {
    }
    frame "AT-DIO-32F" {
    }
    frame "AT-DIO-32HS" {
    }
    frame "AT-DSP2200" {
    }
    frame "AT-GPIB" {
    }
    frame "AT-GPIB/TNT" {
    }
    frame "AT-GPIB/TNT (PnP)" {
    }
    frame "AT-GPIB/TNT+" {
    }
    frame "AT-MIO-16DE-10" {
    }
    frame "AT-MIO-16DH-25" {
    }
    frame "AT-MIO-16DH-9" {
    }
    frame "AT-MIO-16DL-25" {
    }
    frame "AT-MIO-16DL-9" {
    }
    frame "AT-MIO-16E-1" {
    }
    frame "AT-MIO-16E-10" {
    }
    frame "AT-MIO-16E-2" {
    }
    frame "AT-MIO-16F-5" {
    }
    frame "AT-MIO-16H-15" {
    }
    frame "AT-MIO-16H-25" {
    }
    frame "AT-MIO-16H-9" {
    }
    frame "AT-MIO-16L-15" {
    }
    frame "AT-MIO-16L-25" {
    }
    frame "AT-MIO-16L-9" {
    }
    frame "AT-MIO-16X" {
    }
    frame "AT-MIO-16XE-10" {
    }
    frame "AT-MIO-16XE-50" {
    }
    frame "AT-MIO-64E-3" {
    }
    frame "AT-MIO-64F-5" {
    }
    frame "AT-MXI" {
    }
    frame "AT-MXI-2" {
    }
    frame "BNC-2080" {
    }
    frame "BNC-2081" {
    }
    frame "BNC-2082" {
    }
    frame "BNC-2090" {
    }
    frame "BNC-2090A" {
    }
    frame "BNC-2095" {
    }
    frame "BNC-2096" {
    }
    frame "BNC-2110" {
    }
    frame "BNC-2111" {
    }
    frame "BNC-2115" {
    }
    frame "BNC-2120" {
    }
    frame "BNC-2121" {
    }
    frame "BNC-2140" {
    }
    frame "BNC-2142" {
    }
    frame "CAL-4353" {
    }
    frame "CB-100" {
    }
    frame "CB-27" {
    }
    frame "CB-27T" {
    }
    frame "CB-37F-HVD" {
    }
    frame "CB-50" {
    }
    frame "CB-50LC" {
    }
    frame "CB-50LP" {
    }
    frame "CB-68LP" {
    }
    frame "CB-68LPR" {
    }
    frame "CB-68T" {
    }
    frame "CEC USBDAQ/108" {
    }
    frame "CEC USBDAQ/109" {
    }
    frame "CF-6004" {
    }
    frame "CVS-1450" {
    }
    frame "CVS-1451RT" {
    }
    frame "CVS-1454" {
    }
    frame "CVS-1455" {
    }
    frame "CVS-1457RT" {
    }
    frame "CVS-1458RT" {
    }
    frame "CVS-1459RT" {
    }
    frame "CompactRIO PROFINET Slave Module" {
    }
    frame "DAQCard-1200" {
    }
    frame "DAQCard-4050" {
    }
    frame "DAQCard-4350" {
    }
    frame "DAQCard-4502" {
    }
    frame "DAQCard-500" {
    }
    frame "DAQCard-5102" {
    }
    frame "DAQCard-516" {
    }
    frame "DAQCard-5402" {
    }
    frame "DAQCard-6023E" {
    }
    frame "DAQCard-6024E" {
    }
    frame "DAQCard-6034E" {
    }
    frame "DAQCard-6035E" {
    }
    frame "DAQCard-6036E" {
    }
    frame "DAQCard-6062E" {
    }
    frame "DAQCard-6533" {
    }
    frame "DAQCard-6601" {
    }
    frame "DAQCard-6715" {
    }
    frame "DAQCard-6830" {
    }
    frame "DAQCard-700" {
    }
    frame "DAQCard-AI-16E-4" {
    }
    frame "DAQCard-AI-16XE-50" {
    }
    frame "DAQCard-AO-2DC" {
    }
    frame "DAQCard-DIO-24" {
    }
    frame "DAQPad-1200" {
    }
    frame "DAQPad-4350 for USB" {
    }
    frame "DAQPad-4351 for IEEE 1394" {
    }
    frame "DAQPad-4352 for USB" {
    }
    frame "DAQPad-5102" {
    }
    frame "DAQPad-5112 for IEEE 1394" {
    }
    frame "DAQPad-6015 for USB" {
    }
    frame "DAQPad-6015 for USB w/BNC Term" {
    }
    frame "DAQPad-6015 for USB w/Mass Term" {
    }
    frame "DAQPad-6015 for USB w/Screw Term" {
    }
    frame "DAQPad-6016 for USB w/Screw Term" {
    }
    frame "DAQPad-6020E for USB w/BNC Term" {
    }
    frame "DAQPad-6020E for USB w/Mass Term" {
    }
    frame "DAQPad-6024E for USB w/BNC Term" {
    }
    frame "DAQPad-6024E for USB w/Mass Term" {
    }
    frame "DAQPad-6025E for USB w/BNC Term" {
    }
    frame "DAQPad-6025E for USB w/Mass Term" {
    }
    frame "DAQPad-6036E for USB w/BNC Term" {
    }
    frame "DAQPad-6036E for USB w/Mass Term" {
    }
    frame "DAQPad-6052E for Ethernet w/BNC Term" {
    }
    frame "DAQPad-6052E for Ethernet w/Mass Term" {
    }
    frame "DAQPad-6052E for IEEE 1394 w/BNC Term" {
    }
    frame "DAQPad-6052E for IEEE 1394 w/Mass Term" {
    }
    frame "DAQPad-6052E for USB w/BNC Term" {
    }
    frame "DAQPad-6052E for USB w/Mass Term" {
    }
    frame "DAQPad-6070E for IEEE 1394 w/BNC Term" {
    }
    frame "DAQPad-6070E for IEEE 1394 w/Mass Term" {
    }
    frame "DAQPad-6507 for USB" {
    }
    frame "DAQPad-6508 for USB" {
    }
    frame "DAQPad-6533 for IEEE 1394" {
    }
    frame "DAQPad-6713 for IEEE 1394 w/Mass Term" {
    }
    frame "DAQPad-MIO-16XE-50" {
    }
    frame "DAQPad-TB-52" {
    }
    frame "EISA-A2000" {
    }
    frame "EISA-GPIB" {
    }
    frame "ENET-232/2" {
    }
    frame "ENET-232/4" {
    }
    frame "ENET-485/2" {
    }
    frame "ENET-485/4" {
    }
    frame "ENET-7344" {
    }
    frame "ENET-9205" {
    }
    frame "ENET-9205 DSUB" {
    }
    frame "ENET-9206" {
    }
    frame "ENET-9211" {
    }
    frame "ENET-9213" {
    }
    frame "ENET-9215" {
    }
    frame "ENET-9215 BNC" {
    }
    frame "ENET-9219" {
    }
    frame "ENET-9234" {
    }
    frame "ENET-9237" {
    }
    frame "ENET-9421" {
    }
    frame "ENET-9421 DSUB" {
    }
    frame "ENET-9472" {
    }
    frame "ENET-9472 DSUB" {
    }
    frame "ENET-9481" {
    }
    frame "ER-16" {
    }
    frame "ER-8" {
    }
    frame "FP-1000" {
    }
    frame "FP-1001" {
    }
    frame "FP-1300" {
    }
    frame "FP-1600" {
    }
    frame "FP-1601" {
    }
    frame "FP-2000" {
    }
    frame "FP-2010" {
    }
    frame "FP-2015" {
    }
    frame "FP-3000" {
    }
    frame "FP-AI-100" {
    }
    frame "FP-AI-102" {
    }
    frame "FP-AI-110" {
    }
    frame "FP-AI-111" {
    }
    frame "FP-AI-112" {
    }
    frame "FP-AIO-600" {
    }
    frame "FP-AIO-610" {
    }
    frame "FP-AO-200" {
    }
    frame "FP-AO-210" {
    }
    frame "FP-CTR-500" {
    }
    frame "FP-CTR-502" {
    }
    frame "FP-DI-300" {
    }
    frame "FP-DI-301" {
    }
    frame "FP-DI-330" {
    }
    frame "FP-DIO-550" {
    }
    frame "FP-DO-400" {
    }
    frame "FP-DO-401" {
    }
    frame "FP-DO-403" {
    }
    frame "FP-DO-410" {
    }
    frame "FP-PG-522" {
    }
    frame "FP-PWM-520" {
    }
    frame "FP-QUAD-510" {
    }
    frame "FP-RLY-420" {
    }
    frame "FP-RLY-422" {
    }
    frame "FP-RTD-122" {
    }
    frame "FP-RTD-124" {
    }
    frame "FP-SG-140" {
    }
    frame "FP-TB-1 for USB" {
    }
    frame "FP-TC-120" {
    }
    frame "FP-TC-125" {
    }
    frame "FW-7344" {
    }
    frame "GPIB-1394" {
    }
    frame "GPIB-ENET/100" {
    }
    frame "GPIB-PCII" {
    }
    frame "GPIB-PCII/IIA" {
    }
    frame "GPIB-USB" {
    }
    frame "GPIB-USB-A" {
    }
    frame "GPIB-USB-B" {
    }
    frame "GPIB-USB-HS" {
    }
    frame "GPIB-VXI/C" {
    }
    frame "IC-3120" {
    }
    frame "IC-3121" {
    }
    frame "IC-3171" {
    }
    frame "IC-3172" {
    }
    frame "IC-3173" {
    }
    frame "ISC-1780" {
    }
    frame "ISC-1780 (Color)" {
    }
    frame "ISC-1781" {
    }
    frame "ISC-1781 (Color)" {
    }
    frame "ISC-1782" {
    }
    frame "ISC-1782 (Color)" {
    }
    frame "ISC-1783" {
    }
    frame "ISC-1783 (Color)" {
    }
    frame "Lab-PC" {
    }
    frame "Lab-PC+" {
    }
    frame "Lab-PC-1200" {
    }
    frame "Lab-PC-1200AI" {
    }
    frame "MC-DIO-24" {
    }
    frame "MC-DIO-32F" {
    }
    frame "MC-MIO-16H-15" {
    }
    frame "MC-MIO-16H-25" {
    }
    frame "MC-MIO-16L-15" {
    }
    frame "MC-MIO-16L-25" {
    }
    frame "MC-MIO-16L-9" {
    }
    frame "MCC USB-488" {
    }
    frame "NB-MIO-16H-9" {
    }
    frame "NEC-AI-16E-4" {
    }
    frame "NEC-AI-16XE-50" {
    }
    frame "NEC-GPIB/TNT" {
    }
    frame "NEC-GPIB/TNT (PnP)" {
    }
    frame "NEC-MIO-16E-4" {
    }
    frame "NEC-MIO-16XE-50" {
    }
    frame "NET2280" {
    }
    frame "NI 1483" {
    }
    frame "NI 1485" {
    }
    frame "NI 1712" {
    }
    frame "NI 1722" {
    }
    frame "NI 1732" {
    }
    frame "NI 1742" {
    }
    frame "NI 1744" {
    }
    frame "NI 1752" {
    }
    frame "NI 1754" {
    }
    frame "NI 1762" {
    }
    frame "NI 1764" {
    }
    frame "NI 1772" {
    }
    frame "NI 1772C" {
    }
    frame "NI 1774" {
    }
    frame "NI 1774C" {
    }
    frame "NI 1776" {
    }
    frame "NI 1776C" {
    }
    frame "NI 1778" {
    }
    frame "NI 17XX Series Smart Camera" {
    }
    frame "NI 2810" {
    }
    frame "NI 2811" {
    }
    frame "NI 2812" {
    }
    frame "NI 2813" {
    }
    frame "NI 2814" {
    }
    frame "NI 2815" {
    }
    frame "NI 2816" {
    }
    frame "NI 2817" {
    }
    frame "NI 2833" {
    }
    frame "NI 2834" {
    }
    frame "NI 2865" {
    }
    frame "NI 4472 for IEEE 1394" {
    }
    frame "NI 5731" {
    }
    frame "NI 5732" {
    }
    frame "NI 5733" {
    }
    frame "NI 5734" {
    }
    frame "NI 5741" {
    }
    frame "NI 5742" {
    }
    frame "NI 5751" {
    }
    frame "NI 5751B" {
    }
    frame "NI 5752" {
    }
    frame "NI 5752B" {
    }
    frame "NI 5753" {
    }
    frame "NI 5753 (-01) AC" {
    }
    frame "NI 5753 (-02) DC" {
    }
    frame "NI 5761" {
    }
    frame "NI 5771" {
    }
    frame "NI 5772" {
    }
    frame "NI 5781" {
    }
    frame "NI 5782" {
    }
    frame "NI 5782 (DC)" {
    }
    frame "NI 5783" {
    }
    frame "NI 5791" {
    }
    frame "NI 5792" {
    }
    frame "NI 5793" {
    }
    frame "NI 6224 for Ethernet w/BNC Term" {
    }
    frame "NI 6224 for Ethernet w/Mass Term" {
    }
    frame "NI 6224 for Ethernet w/SCXI Term" {
    }
    frame "NI 6225 for Ethernet" {
    }
    frame "NI 6226 for Ethernet" {
    }
    frame "NI 6581" {
    }
    frame "NI 6581B" {
    }
    frame "NI 6583" {
    }
    frame "NI 6584" {
    }
    frame "NI 6585" {
    }
    frame "NI 6585B" {
    }
    frame "NI 6587" {
    }
    frame "NI 6588" {
    }
    frame "NI 6589" {
    }
    frame "NI 7451" {
    }
    frame "NI 9145" {
    }
    frame "NI 9146" {
    }
    frame "NI 9147" {
    }
    frame "NI 9148" {
    }
    frame "NI 9149" {
    }
    frame "NI 9154" {
    }
    frame "NI 9155" {
    }
    frame "NI 9157" {
    }
    frame "NI 9159" {
    }
    frame "NI 9201" {
    }
    frame "NI 9201 D-Sub" {
    }
    frame "NI 9201 cRIO" {
    }
    frame "NI 9203" {
    }
    frame "NI 9203 cRIO" {
    }
    frame "NI 9205" {
    }
    frame "NI 9205 (DSUB)" {
    }
    frame "NI 9205 D-Sub" {
    }
    frame "NI 9205 cRIO" {
    }
    frame "NI 9206" {
    }
    frame "NI 9206 cRIO" {
    }
    frame "NI 9207" {
    }
    frame "NI 9208" {
    }
    frame "NI 9209" {
    }
    frame "NI 9210" {
    }
    frame "NI 9211" {
    }
    frame "NI 9211 cRIO" {
    }
    frame "NI 9212" {
    }
    frame "NI 9213" {
    }
    frame "NI 9214" {
    }
    frame "NI 9215" {
    }
    frame "NI 9215 (BNC)" {
    }
    frame "NI 9215 BNC" {
    }
    frame "NI 9215 cRIO" {
    }
    frame "NI 9215E" {
    }
    frame "NI 9216" {
    }
    frame "NI 9217" {
    }
    frame "NI 9217 cRIO" {
    }
    frame "NI 9218" {
    }
    frame "NI 9219" {
    }
    frame "NI 9219 LEMO" {
    }
    frame "NI 9219 cRIO" {
    }
    frame "NI 9219E" {
    }
    frame "NI 9220" {
    }
    frame "NI 9220 cDAQ" {
    }
    frame "NI 9221" {
    }
    frame "NI 9221 (DSUB)" {
    }
    frame "NI 9221 (DSUB) cRIO" {
    }
    frame "NI 9221 cRIO" {
    }
    frame "NI 9222" {
    }
    frame "NI 9223" {
    }
    frame "NI 9223 cDAQ" {
    }
    frame "NI 9224" {
    }
    frame "NI 9225" {
    }
    frame "NI 9225 cRIO" {
    }
    frame "NI 9226" {
    }
    frame "NI 9227" {
    }
    frame "NI 9228" {
    }
    frame "NI 9229" {
    }
    frame "NI 9229 (BNC)" {
    }
    frame "NI 9229 BNC" {
    }
    frame "NI 9229 cRIO" {
    }
    frame "NI 9230" {
    }
    frame "NI 9230 BNC cDAQ" {
    }
    frame "NI 9232" {
    }
    frame "NI 9232 BNC cDAQ" {
    }
    frame "NI 9232 cDAQ" {
    }
    frame "NI 9232E" {
    }
    frame "NI 9233" {
    }
    frame "NI 9234" {
    }
    frame "NI 9234B" {
    }
    frame "NI 9234E" {
    }
    frame "NI 9235" {
    }
    frame "NI 9236" {
    }
    frame "NI 9237" {
    }
    frame "NI 9237 cRIO" {
    }
    frame "NI 9237 with D-Sub" {
    }
    frame "NI 9238" {
    }
    frame "NI 9239" {
    }
    frame "NI 9239 (BNC)" {
    }
    frame "NI 9239 BNC" {
    }
    frame "NI 9239 cRIO" {
    }
    frame "NI 9242" {
    }
    frame "NI 9244" {
    }
    frame "NI 9246" {
    }
    frame "NI 9247" {
    }
    frame "NI 9250" {
    }
    frame "NI 9251" {
    }
    frame "NI 9251 Mini XLR cDAQ" {
    }
    frame "NI 9260" {
    }
    frame "NI 9263" {
    }
    frame "NI 9263 (BNC)" {
    }
    frame "NI 9263 cRIO" {
    }
    frame "NI 9264" {
    }
    frame "NI 9264 D-sub" {
    }
    frame "NI 9264 cRIO" {
    }
    frame "NI 9265" {
    }
    frame "NI 9265 cRIO" {
    }
    frame "NI 9265E" {
    }
    frame "NI 9266" {
    }
    frame "NI 9269" {
    }
    frame "NI 9344" {
    }
    frame "NI 9361" {
    }
    frame "NI 9375" {
    }
    frame "NI 9375 (DSUB)" {
    }
    frame "NI 9381 DSUB" {
    }
    frame "NI 9401" {
    }
    frame "NI 9401 cRIO" {
    }
    frame "NI 9402" {
    }
    frame "NI 9402 cRIO" {
    }
    frame "NI 9403" {
    }
    frame "NI 9403 cRIO" {
    }
    frame "NI 9411" {
    }
    frame "NI 9411 cRIO" {
    }
    frame "NI 9421" {
    }
    frame "NI 9421 (DSUB)" {
    }
    frame "NI 9421 D-Sub" {
    }
    frame "NI 9421 cRIO" {
    }
    frame "NI 9422" {
    }
    frame "NI 9422 cRIO" {
    }
    frame "NI 9423" {
    }
    frame "NI 9423 cRIO" {
    }
    frame "NI 9425" {
    }
    frame "NI 9425 cRIO" {
    }
    frame "NI 9426" {
    }
    frame "NI 9426 cRIO" {
    }
    frame "NI 9435" {
    }
    frame "NI 9435 cRIO" {
    }
    frame "NI 9436" {
    }
    frame "NI 9437" {
    }
    frame "NI 9467" {
    }
    frame "NI 9469" {
    }
    frame "NI 9472" {
    }
    frame "NI 9472 (DSUB)" {
    }
    frame "NI 9472 D-Sub" {
    }
    frame "NI 9472 cRIO" {
    }
    frame "NI 9474" {
    }
    frame "NI 9474 cRIO" {
    }
    frame "NI 9475" {
    }
    frame "NI 9476" {
    }
    frame "NI 9476 cRIO" {
    }
    frame "NI 9477" {
    }
    frame "NI 9477 cRIO" {
    }
    frame "NI 9478 cRIO" {
    }
    frame "NI 9481" {
    }
    frame "NI 9481 cRIO" {
    }
    frame "NI 9481E" {
    }
    frame "NI 9482" {
    }
    frame "NI 9485" {
    }
    frame "NI 9485 cRIO" {
    }
    frame "NI 9501" {
    }
    frame "NI 9502" {
    }
    frame "NI 9503" {
    }
    frame "NI 9505" {
    }
    frame "NI 9512" {
    }
    frame "NI 9514" {
    }
    frame "NI 9516" {
    }
    frame "NI 9770" {
    }
    frame "NI 9775" {
    }
    frame "NI 9792" {
    }
    frame "NI 9795" {
    }
    frame "NI 9802 cRIO" {
    }
    frame "NI 9841" {
    }
    frame "NI 9853" {
    }
    frame "NI 9860" {
    }
    frame "NI 9861" {
    }
    frame "NI 9862" {
    }
    frame "NI 9866" {
    }
    frame "NI 9870 cRIO" {
    }
    frame "NI 9870E" {
    }
    frame "NI 9871 cRIO" {
    }
    frame "NI 9871E" {
    }
    frame "NI Bluetooth Toolkit" {
    }
    frame "NI CAN Interfaces (Series 2)" {
    }
    frame "NI CVS-1450 Series" {
    }
    frame "NI DeviceNet Interfaces" {
    }
    frame "NI ELVIS II" {
    }
    frame "NI ELVIS II+" {
    }
    frame "NI EVS-1460 Series" {
    }
    frame "NI ExpressCard-8360" {
    }
    frame "NI ExpressCard-8420/2" {
    }
    frame "NI ExpressCard-8421/2" {
    }
    frame "NI ExpressCard-GPIB" {
    }
    frame "NI PCI-8511 CAN/LS1" {
    }
    frame "NI PCI-8511 CAN/LS2" {
    }
    frame "NI PCI-8512 CAN/HS1" {
    }
    frame "NI PCI-8512 CAN/HS2" {
    }
    frame "NI PCI-8513 CAN/XS1" {
    }
    frame "NI PCI-8513 CAN/XS2" {
    }
    frame "NI PCI-8516 LIN/2" {
    }
    frame "NI PCI-8517 FlexRay2" {
    }
    frame "NI PCIe-1427" {
    }
    frame "NI PCIe-1429" {
    }
    frame "NI PCIe-1430" {
    }
    frame "NI PCIe-1433" {
    }
    frame "NI PCIe-4065" {
    }
    frame "NI PCIe-5122" {
    }
    frame "NI PCIe-5142" {
    }
    frame "NI PCIe-6250" {
    }
    frame "NI PCIe-6251" {
    }
    frame "NI PCIe-6259" {
    }
    frame "NI PCIe-6344R" {
    }
    frame "NI PCIe-6346R" {
    }
    frame "NI PCIe-6509" {
    }
    frame "NI PCIe-6535" {
    }
    frame "NI PCIe-6536" {
    }
    frame "NI PCIe-6537" {
    }
    frame "NI PCIe-6542" {
    }
    frame "NI PCIe-6552" {
    }
    frame "NI PCIe-8231" {
    }
    frame "NI PCIe-8235" {
    }
    frame "NI PCIe-8253" {
    }
    frame "NI PCIe-8255R" {
    }
    frame "NI PCIe-GPIB" {
    }
    frame "NI PXI-4110" {
    }
    frame "NI PXI-4130" {
    }
    frame "NI PXI-4131A" {
    }
    frame "NI PXI-4132" {
    }
    frame "NI PXI-8511 CAN/LS1" {
    }
    frame "NI PXI-8511 CAN/LS2" {
    }
    frame "NI PXI-8512 CAN/HS1" {
    }
    frame "NI PXI-8512 CAN/HS2" {
    }
    frame "NI PXI-8513 CAN/XS1" {
    }
    frame "NI PXI-8513 CAN/XS2" {
    }
    frame "NI PXI-8516 LIN/2" {
    }
    frame "NI PXI-8517 FlexRay2" {
    }
    frame "NI PXIe-1062Q" {
    }
    frame "NI PXIe-1065" {
    }
    frame "NI PXIe-1436" {
    }
    frame "NI PXIe-1491" {
    }
    frame "NI PXIe-4112" {
    }
    frame "NI PXIe-4113" {
    }
    frame "NI PXIe-4136" {
    }
    frame "NI PXIe-4137" {
    }
    frame "NI PXIe-4138" {
    }
    frame "NI PXIe-4139" {
    }
    frame "NI PXIe-4140" {
    }
    frame "NI PXIe-4141" {
    }
    frame "NI PXIe-4142" {
    }
    frame "NI PXIe-4143" {
    }
    frame "NI PXIe-4144" {
    }
    frame "NI PXIe-4145" {
    }
    frame "NI PXIe-4154" {
    }
    frame "NI PXIe-4496" {
    }
    frame "NI PXIe-4498" {
    }
    frame "NI PXIe-5122" {
    }
    frame "NI PXIe-5142" {
    }
    frame "NI PXIe-5421" {
    }
    frame "NI PXIe-5422" {
    }
    frame "NI PXIe-5442" {
    }
    frame "NI PXIe-5450" {
    }
    frame "NI PXIe-5451" {
    }
    frame "NI PXIe-5452" {
    }
    frame "NI PXIe-5453" {
    }
    frame "NI PXIe-5455" {
    }
    frame "NI PXIe-5602" {
    }
    frame "NI PXIe-5612" {
    }
    frame "NI PXIe-5622" {
    }
    frame "NI PXIe-6251" {
    }
    frame "NI PXIe-6259" {
    }
    frame "NI PXIe-6535" {
    }
    frame "NI PXIe-6536" {
    }
    frame "NI PXIe-6537" {
    }
    frame "NI PXIe-6542" {
    }
    frame "NI PXIe-6552" {
    }
    frame "NI PXIe-8103" {
    }
    frame "NI PXIe-8105" {
    }
    frame "NI PXIe-8106" {
    }
    frame "NI PXIe-8130" {
    }
    frame "NI PXIe-8131" {
    }
    frame "NI PXIe-8234" {
    }
    frame "NI SoftMotion Controller for CANopen" {
    }
    frame "NI SoftMotion Controller for IEEE 1394" {
    }
    frame "NI TBX-2808" {
    }
    frame "NI USB 7845R" {
    }
    frame "NI USB 7845R OEM" {
    }
    frame "NI USB 7846R OEM" {
    }
    frame "NI USB-6341" {
    }
    frame "NI USB-6341 OEM" {
    }
    frame "NI USB-6343" {
    }
    frame "NI USB-6343 OEM" {
    }
    frame "NI USB-6351" {
    }
    frame "NI USB-6353" {
    }
    frame "NI USB-6356 (32 MS) (Screw Terminal)" {
    }
    frame "NI USB-6356 (32MS)" {
    }
    frame "NI USB-6356 (32MS) OEM" {
    }
    frame "NI USB-6356 (64 MS) (Screw Terminal)" {
    }
    frame "NI USB-6356 (64MS)" {
    }
    frame "NI USB-6361" {
    }
    frame "NI USB-6361 OEM" {
    }
    frame "NI USB-6363" {
    }
    frame "NI USB-6363 OEM" {
    }
    frame "NI USB-6366 (32 MS) (Screw Terminal)" {
    }
    frame "NI USB-6366 (32MS)" {
    }
    frame "NI USB-6366 (64 MS) (Screw Terminal)" {
    }
    frame "NI USB-6366 (64MS)" {
    }
    frame "NI USB-6366 (64MS) OEM" {
    }
    frame "NI USB-7846R" {
    }
    frame "NI USB-7855R" {
    }
    frame "NI USB-7855R OEM" {
    }
    frame "NI USB-7856R" {
    }
    frame "NI USB-7856R OEM" {
    }
    frame "NI USB-TC01" {
    }
    frame "NI USRP-2944R" {
    }
    frame "NI USRP-2954R" {
    }
    frame "NI WSN-3202" {
    }
    frame "NI WSN-3202 (programmable)" {
    }
    frame "NI WSN-3212" {
    }
    frame "NI WSN-3212 (programmable)" {
    }
    frame "NI WSN-3214" {
    }
    frame "NI WSN-3214 LV" {
    }
    frame "NI WSN-3226" {
    }
    frame "NI WSN-3226 (programmable)" {
    }
    frame "NI WSN-3230" {
    }
    frame "NI WSN-3231" {
    }
    frame "NI WSN-3234" {
    }
    frame "NI WSN-3234 LV" {
    }
    frame "NI WSN-9791" {
    }
    frame "NI WSN-9792 OEM" {
    }
    frame "NI myDAQ" {
    }
    frame "NI myDAQ Hardware" {
    }
    frame "NI myRIO" {
    }
    frame "NI roboRIO" {
    }
    frame "NI-1702" {
    }
    frame "NI-7931" {
    }
    frame "NI-7932" {
    }
    frame "NI-7935" {
    }
    frame "NI-9852" {
    }
    frame "NI-IMAQ for IEEE 1394 Cameras" {
    }
    frame "OEM USB-7931R" {
    }
    frame "OEM USB-7932R" {
    }
    frame "OEM USB-7933R" {
    }
    frame "PC-4350" {
    }
    frame "PC-516" {
    }
    frame "PC-AO-2DC" {
    }
    frame "PC-DIO-24" {
    }
    frame "PC-DIO-96" {
    }
    frame "PC-DIO-96PnP" {
    }
    frame "PC-FlexMotion-6C" {
    }
    frame "PC-LPM-16" {
    }
    frame "PC-LPM-16PnP" {
    }
    frame "PC-OPDIO-16" {
    }
    frame "PC-Servo-1P" {
    }
    frame "PC-Servo-2A" {
    }
    frame "PC-Servo-4A" {
    }
    frame "PC-Step-2CX" {
    }
    frame "PC-Step-2OX" {
    }
    frame "PC-Step-4CX" {
    }
    frame "PC-Step-4OX" {
    }
    frame "PC-TIO-10" {
    }
    frame "PCI-1200" {
    }
    frame "PCI-1405" {
    }
    frame "PCI-1407" {
    }
    frame "PCI-1408" {
    }
    frame "PCI-1409" {
    }
    frame "PCI-1410" {
    }
    frame "PCI-1411" {
    }
    frame "PCI-1412" {
    }
    frame "PCI-1413" {
    }
    frame "PCI-1422" {
    }
    frame "PCI-1423" {
    }
    frame "PCI-1424" {
    }
    frame "PCI-1426" {
    }
    frame "PCI-1428" {
    }
    frame "PCI-1588" {
    }
    frame "PCI-232/16" {
    }
    frame "PCI-232/2" {
    }
    frame "PCI-232/4" {
    }
    frame "PCI-232/8" {
    }
    frame "PCI-232I/2" {
    }
    frame "PCI-232I/4" {
    }
    frame "PCI-4021" {
    }
    frame "PCI-4060" {
    }
    frame "PCI-4065" {
    }
    frame "PCI-4070" {
    }
    frame "PCI-4351" {
    }
    frame "PCI-4451" {
    }
    frame "PCI-4452" {
    }
    frame "PCI-4453" {
    }
    frame "PCI-4454" {
    }
    frame "PCI-4461" {
    }
    frame "PCI-4462" {
    }
    frame "PCI-4472" {
    }
    frame "PCI-4472B" {
    }
    frame "PCI-4474" {
    }
    frame "PCI-4551" {
    }
    frame "PCI-4552" {
    }
    frame "PCI-485/2" {
    }
    frame "PCI-485/4" {
    }
    frame "PCI-485/8" {
    }
    frame "PCI-485I/2" {
    }
    frame "PCI-485I/4" {
    }
    frame "PCI-488" {
    }
    frame "PCI-488LP" {
    }
    frame "PCI-5102" {
    }
    frame "PCI-5104" {
    }
    frame "PCI-5105" {
    }
    frame "PCI-5112" {
    }
    frame "PCI-5114" {
    }
    frame "PCI-5122" {
    }
    frame "PCI-5124" {
    }
    frame "PCI-5142" {
    }
    frame "PCI-5152" {
    }
    frame "PCI-5153" {
    }
    frame "PCI-5154" {
    }
    frame "PCI-5401" {
    }
    frame "PCI-5402" {
    }
    frame "PCI-5406" {
    }
    frame "PCI-5411" {
    }
    frame "PCI-5412" {
    }
    frame "PCI-5420" {
    }
    frame "PCI-5421" {
    }
    frame "PCI-5422" {
    }
    frame "PCI-5431" {
    }
    frame "PCI-5640R" {
    }
    frame "PCI-5911" {
    }
    frame "PCI-5922" {
    }
    frame "PCI-5922EX" {
    }
    frame "PCI-6010" {
    }
    frame "PCI-6011E" {
    }
    frame "PCI-6013" {
    }
    frame "PCI-6014" {
    }
    frame "PCI-6023E" {
    }
    frame "PCI-6024E" {
    }
    frame "PCI-6025E" {
    }
    frame "PCI-6030E" {
    }
    frame "PCI-6031E" {
    }
    frame "PCI-6032E" {
    }
    frame "PCI-6033E" {
    }
    frame "PCI-6034E" {
    }
    frame "PCI-6035E" {
    }
    frame "PCI-6036E" {
    }
    frame "PCI-6040E (PCI-MIO-16E-4)" {
    }
    frame "PCI-6052E" {
    }
    frame "PCI-6053E" {
    }
    frame "PCI-6070E" {
    }
    frame "PCI-6071E" {
    }
    frame "PCI-6110" {
    }
    frame "PCI-6111" {
    }
    frame "PCI-6115" {
    }
    frame "PCI-6120" {
    }
    frame "PCI-6122" {
    }
    frame "PCI-6123" {
    }
    frame "PCI-6132" {
    }
    frame "PCI-6133" {
    }
    frame "PCI-6143" {
    }
    frame "PCI-6154" {
    }
    frame "PCI-6220" {
    }
    frame "PCI-6221" {
    }
    frame "PCI-6221 (37-Pin)" {
    }
    frame "PCI-6222" {
    }
    frame "PCI-6224" {
    }
    frame "PCI-6225" {
    }
    frame "PCI-6229" {
    }
    frame "PCI-6230" {
    }
    frame "PCI-6232" {
    }
    frame "PCI-6233" {
    }
    frame "PCI-6236" {
    }
    frame "PCI-6238" {
    }
    frame "PCI-6239" {
    }
    frame "PCI-6250" {
    }
    frame "PCI-6251" {
    }
    frame "PCI-6254" {
    }
    frame "PCI-6255" {
    }
    frame "PCI-6259" {
    }
    frame "PCI-6280" {
    }
    frame "PCI-6281" {
    }
    frame "PCI-6284" {
    }
    frame "PCI-6289" {
    }
    frame "PCI-6503" {
    }
    frame "PCI-6504" {
    }
    frame "PCI-6505" {
    }
    frame "PCI-6509" {
    }
    frame "PCI-6510" {
    }
    frame "PCI-6511" {
    }
    frame "PCI-6512" {
    }
    frame "PCI-6513" {
    }
    frame "PCI-6514" {
    }
    frame "PCI-6515" {
    }
    frame "PCI-6516" {
    }
    frame "PCI-6517" {
    }
    frame "PCI-6518" {
    }
    frame "PCI-6519" {
    }
    frame "PCI-6520" {
    }
    frame "PCI-6521" {
    }
    frame "PCI-6525" {
    }
    frame "PCI-6526" {
    }
    frame "PCI-6527" {
    }
    frame "PCI-6528" {
    }
    frame "PCI-6533" {
    }
    frame "PCI-6534" {
    }
    frame "PCI-6541" {
    }
    frame "PCI-6542" {
    }
    frame "PCI-6551" {
    }
    frame "PCI-6552" {
    }
    frame "PCI-6561" {
    }
    frame "PCI-6562" {
    }
    frame "PCI-6601" {
    }
    frame "PCI-6602" {
    }
    frame "PCI-6608" {
    }
    frame "PCI-6610" {
    }
    frame "PCI-6624" {
    }
    frame "PCI-6703" {
    }
    frame "PCI-6704" {
    }
    frame "PCI-6711" {
    }
    frame "PCI-6713" {
    }
    frame "PCI-6722" {
    }
    frame "PCI-6723" {
    }
    frame "PCI-6731" {
    }
    frame "PCI-6733" {
    }
    frame "PCI-6810" {
    }
    frame "PCI-7030/6030E" {
    }
    frame "PCI-7030/6040E" {
    }
    frame "PCI-7040/6040E" {
    }
    frame "PCI-7041/6040E" {
    }
    frame "PCI-716" {
    }
    frame "PCI-7314" {
    }
    frame "PCI-7324" {
    }
    frame "PCI-7330" {
    }
    frame "PCI-7332" {
    }
    frame "PCI-7334" {
    }
    frame "PCI-7340" {
    }
    frame "PCI-7342" {
    }
    frame "PCI-7344" {
    }
    frame "PCI-7346" {
    }
    frame "PCI-7350" {
    }
    frame "PCI-7390" {
    }
    frame "PCI-7414" {
    }
    frame "PCI-7811R" {
    }
    frame "PCI-7813R" {
    }
    frame "PCI-7830R" {
    }
    frame "PCI-7831R" {
    }
    frame "PCI-7833R" {
    }
    frame "PCI-7841R" {
    }
    frame "PCI-7842R" {
    }
    frame "PCI-7851R" {
    }
    frame "PCI-7852R" {
    }
    frame "PCI-7853R" {
    }
    frame "PCI-8215" {
    }
    frame "PCI-8252" {
    }
    frame "PCI-8254R" {
    }
    frame "PCI-8320" {
    }
    frame "PCI-8410/2" {
    }
    frame "PCI-8430/16" {
    }
    frame "PCI-8430/2" {
    }
    frame "PCI-8430/4" {
    }
    frame "PCI-8430/8" {
    }
    frame "PCI-8431/2" {
    }
    frame "PCI-8431/4" {
    }
    frame "PCI-8431/8" {
    }
    frame "PCI-8432/2" {
    }
    frame "PCI-8432/4" {
    }
    frame "PCI-8433/2" {
    }
    frame "PCI-8433/4" {
    }
    frame "PCI-CAN" {
    }
    frame "PCI-CAN (DNET)" {
    }
    frame "PCI-CAN Series 2" {
    }
    frame "PCI-CAN/2" {
    }
    frame "PCI-CAN/2 Series 2" {
    }
    frame "PCI-CAN/DS" {
    }
    frame "PCI-CAN/DS Series 2" {
    }
    frame "PCI-CAN/LS" {
    }
    frame "PCI-CAN/LS Series 2" {
    }
    frame "PCI-CAN/LS2" {
    }
    frame "PCI-CAN/LS2 Series 2" {
    }
    frame "PCI-CAN/SW Series 2" {
    }
    frame "PCI-CAN/SW2 Series 2" {
    }
    frame "PCI-CAN/XS Series 2" {
    }
    frame "PCI-CAN/XS2 Series 2" {
    }
    frame "PCI-DIO-32HS-T" {
    }
    frame "PCI-DIO-96" {
    }
    frame "PCI-FBUS" {
    }
    frame "PCI-FBUS/2" {
    }
    frame "PCI-FlexMotion-6C" {
    }
    frame "PCI-GPIB" {
    }
    frame "PCI-GPIB+" {
    }
    frame "PCI-MXI-2" {
    }
    frame "PCI-MXI-2 Universal" {
    }
    frame "PCI-Servo-2A" {
    }
    frame "PCI-Servo-4A" {
    }
    frame "PCI-Step-2CX" {
    }
    frame "PCI-Step-2OX" {
    }
    frame "PCI-Step-4CX" {
    }
    frame "PCI-Step-4OX" {
    }
    frame "PCIe-1433R" {
    }
    frame "PCIe-1434R" {
    }
    frame "PCIe-1435R" {
    }
    frame "PCIe-1436R" {
    }
    frame "PCIe-1473R" {
    }
    frame "PCIe-1473R-LX110" {
    }
    frame "PCIe-1474R" {
    }
    frame "PCIe-1475R" {
    }
    frame "PCIe-1476R" {
    }
    frame "PCIe-6320" {
    }
    frame "PCIe-6321" {
    }
    frame "PCIe-6323" {
    }
    frame "PCIe-6326" {
    }
    frame "PCIe-6341" {
    }
    frame "PCIe-6343" {
    }
    frame "PCIe-6346" {
    }
    frame "PCIe-6351" {
    }
    frame "PCIe-6353" {
    }
    frame "PCIe-6356" {
    }
    frame "PCIe-6361" {
    }
    frame "PCIe-6363" {
    }
    frame "PCIe-6612" {
    }
    frame "PCIe-8233" {
    }
    frame "PCIe-8236" {
    }
    frame "PCIe-8237R" {
    }
    frame "PCIe-8242" {
    }
    frame "PCIe-8244" {
    }
    frame "PCIe-8430/16" {
    }
    frame "PCIe-8430/8" {
    }
    frame "PCIe-8431/16" {
    }
    frame "PCIe-8431/8" {
    }
    frame "PCIe-GPIB+" {
    }
    frame "PCMCIA-232" {
    }
    frame "PCMCIA-232 921.6k" {
    }
    frame "PCMCIA-232/2" {
    }
    frame "PCMCIA-232/2 921.6k" {
    }
    frame "PCMCIA-232/4" {
    }
    frame "PCMCIA-485" {
    }
    frame "PCMCIA-485 921.6k" {
    }
    frame "PCMCIA-485/2" {
    }
    frame "PCMCIA-485/2 921.6k" {
    }
    frame "PCMCIA-6024E" {
    }
    frame "PCMCIA-6036E" {
    }
    frame "PCMCIA-6062E" {
    }
    frame "PCMCIA-CAN" {
    }
    frame "PCMCIA-CAN (DNET)" {
    }
    frame "PCMCIA-CAN Series 2" {
    }
    frame "PCMCIA-CAN/2" {
    }
    frame "PCMCIA-CAN/2 Series 2" {
    }
    frame "PCMCIA-CAN/LS" {
    }
    frame "PCMCIA-CAN/LS2" {
    }
    frame "PCMCIA-FBUS" {
    }
    frame "PCMCIA-FBUS Series 2" {
    }
    frame "PCMCIA-FBUS/2" {
    }
    frame "PCMCIA-FBUS/2 Series 2" {
    }
    frame "PCMCIA-GPIB" {
    }
    frame "PCMCIA-GPIB+" {
    }
    frame "PMC-GPIB" {
    }
    frame "PSH32-TC6" {
    }
    frame "PXI-1010" {
    }
    frame "PXI-1011" {
    }
    frame "PXI-1033" {
    }
    frame "PXI-1044" {
    }
    frame "PXI-1045" {
    }
    frame "PXI-1050" {
    }
    frame "PXI-1052" {
    }
    frame "PXI-1056" {
    }
    frame "PXI-1405" {
    }
    frame "PXI-1407" {
    }
    frame "PXI-1408" {
    }
    frame "PXI-1409" {
    }
    frame "PXI-1411" {
    }
    frame "PXI-1412" {
    }
    frame "PXI-1413" {
    }
    frame "PXI-1422" {
    }
    frame "PXI-1423" {
    }
    frame "PXI-1424" {
    }
    frame "PXI-1428" {
    }
    frame "PXI-1588" {
    }
    frame "PXI-2501" {
    }
    frame "PXI-2503" {
    }
    frame "PXI-2510" {
    }
    frame "PXI-2512" {
    }
    frame "PXI-2514" {
    }
    frame "PXI-2515" {
    }
    frame "PXI-2520" {
    }
    frame "PXI-2521" {
    }
    frame "PXI-2522" {
    }
    frame "PXI-2523" {
    }
    frame "PXI-2527" {
    }
    frame "PXI-2528" {
    }
    frame "PXI-2529" {
    }
    frame "PXI-2530" {
    }
    frame "PXI-2531" {
    }
    frame "PXI-2532" {
    }
    frame "PXI-2533" {
    }
    frame "PXI-2534" {
    }
    frame "PXI-2535" {
    }
    frame "PXI-2536" {
    }
    frame "PXI-2537" {
    }
    frame "PXI-2538" {
    }
    frame "PXI-2540" {
    }
    frame "PXI-2541" {
    }
    frame "PXI-2542" {
    }
    frame "PXI-2543" {
    }
    frame "PXI-2544" {
    }
    frame "PXI-2545" {
    }
    frame "PXI-2546" {
    }
    frame "PXI-2547" {
    }
    frame "PXI-2548" {
    }
    frame "PXI-2549" {
    }
    frame "PXI-2554" {
    }
    frame "PXI-2555" {
    }
    frame "PXI-2556" {
    }
    frame "PXI-2557" {
    }
    frame "PXI-2558" {
    }
    frame "PXI-2559" {
    }
    frame "PXI-2564" {
    }
    frame "PXI-2565" {
    }
    frame "PXI-2566" {
    }
    frame "PXI-2567" {
    }
    frame "PXI-2568" {
    }
    frame "PXI-2569" {
    }
    frame "PXI-2570" {
    }
    frame "PXI-2571" {
    }
    frame "PXI-2575" {
    }
    frame "PXI-2576" {
    }
    frame "PXI-2584" {
    }
    frame "PXI-2585" {
    }
    frame "PXI-2586" {
    }
    frame "PXI-2590" {
    }
    frame "PXI-2591" {
    }
    frame "PXI-2593" {
    }
    frame "PXI-2594" {
    }
    frame "PXI-2595" {
    }
    frame "PXI-2596" {
    }
    frame "PXI-2597" {
    }
    frame "PXI-2598" {
    }
    frame "PXI-2599" {
    }
    frame "PXI-2720" {
    }
    frame "PXI-2722" {
    }
    frame "PXI-2796" {
    }
    frame "PXI-2797" {
    }
    frame "PXI-2798" {
    }
    frame "PXI-2799" {
    }
    frame "PXI-2810" {
    }
    frame "PXI-2811" {
    }
    frame "PXI-2812" {
    }
    frame "PXI-2813" {
    }
    frame "PXI-2814" {
    }
    frame "PXI-2815" {
    }
    frame "PXI-2816" {
    }
    frame "PXI-2817" {
    }
    frame "PXI-2833" {
    }
    frame "PXI-2834" {
    }
    frame "PXI-2865" {
    }
    frame "PXI-4021" {
    }
    frame "PXI-4022" {
    }
    frame "PXI-4060" {
    }
    frame "PXI-4065" {
    }
    frame "PXI-4070" {
    }
    frame "PXI-4071" {
    }
    frame "PXI-4072" {
    }
    frame "PXI-4130SL" {
    }
    frame "PXI-4170" {
    }
    frame "PXI-4200" {
    }
    frame "PXI-4204" {
    }
    frame "PXI-4220" {
    }
    frame "PXI-4224" {
    }
    frame "PXI-4225" {
    }
    frame "PXI-4351" {
    }
    frame "PXI-4411" {
    }
    frame "PXI-4461" {
    }
    frame "PXI-4461 eHM" {
    }
    frame "PXI-4462" {
    }
    frame "PXI-4462 eHM" {
    }
    frame "PXI-4472" {
    }
    frame "PXI-4472B" {
    }
    frame "PXI-4474" {
    }
    frame "PXI-4492" {
    }
    frame "PXI-4494" {
    }
    frame "PXI-4495" {
    }
    frame "PXI-4496" {
    }
    frame "PXI-4498" {
    }
    frame "PXI-4551" {
    }
    frame "PXI-4552" {
    }
    frame "PXI-485/8" {
    }
    frame "PXI-5102" {
    }
    frame "PXI-5104" {
    }
    frame "PXI-5105" {
    }
    frame "PXI-5112" {
    }
    frame "PXI-5114" {
    }
    frame "PXI-5122" {
    }
    frame "PXI-5124" {
    }
    frame "PXI-5142" {
    }
    frame "PXI-5152" {
    }
    frame "PXI-5153" {
    }
    frame "PXI-5154" {
    }
    frame "PXI-5401" {
    }
    frame "PXI-5402" {
    }
    frame "PXI-5404" {
    }
    frame "PXI-5406" {
    }
    frame "PXI-5411" {
    }
    frame "PXI-5412" {
    }
    frame "PXI-5420" {
    }
    frame "PXI-5421" {
    }
    frame "PXI-5422" {
    }
    frame "PXI-5431" {
    }
    frame "PXI-5433" {
    }
    frame "PXI-5441" {
    }
    frame "PXI-5600" {
    }
    frame "PXI-5610" {
    }
    frame "PXI-5620" {
    }
    frame "PXI-5621" {
    }
    frame "PXI-5650" {
    }
    frame "PXI-5651" {
    }
    frame "PXI-5652" {
    }
    frame "PXI-5653" {
    }
    frame "PXI-5660" {
    }
    frame "PXI-5661" {
    }
    frame "PXI-5670" {
    }
    frame "PXI-5671" {
    }
    frame "PXI-5690" {
    }
    frame "PXI-5691" {
    }
    frame "PXI-5695" {
    }
    frame "PXI-5900" {
    }
    frame "PXI-5911" {
    }
    frame "PXI-5922" {
    }
    frame "PXI-5922EX" {
    }
    frame "PXI-6011E" {
    }
    frame "PXI-6023E" {
    }
    frame "PXI-6024E" {
    }
    frame "PXI-6025E" {
    }
    frame "PXI-6030E" {
    }
    frame "PXI-6031E" {
    }
    frame "PXI-6032E" {
    }
    frame "PXI-6033E" {
    }
    frame "PXI-6035E" {
    }
    frame "PXI-6040E" {
    }
    frame "PXI-6052E" {
    }
    frame "PXI-6053E" {
    }
    frame "PXI-6070E" {
    }
    frame "PXI-6071E" {
    }
    frame "PXI-6115" {
    }
    frame "PXI-6120" {
    }
    frame "PXI-6122" {
    }
    frame "PXI-6123" {
    }
    frame "PXI-6132" {
    }
    frame "PXI-6133" {
    }
    frame "PXI-6143" {
    }
    frame "PXI-6220" {
    }
    frame "PXI-6221" {
    }
    frame "PXI-6222" {
    }
    frame "PXI-6224" {
    }
    frame "PXI-6225" {
    }
    frame "PXI-6229" {
    }
    frame "PXI-6230" {
    }
    frame "PXI-6232" {
    }
    frame "PXI-6233" {
    }
    frame "PXI-6236" {
    }
    frame "PXI-6238" {
    }
    frame "PXI-6239" {
    }
    frame "PXI-6250" {
    }
    frame "PXI-6251" {
    }
    frame "PXI-6254" {
    }
    frame "PXI-6255" {
    }
    frame "PXI-6259" {
    }
    frame "PXI-6280" {
    }
    frame "PXI-6281" {
    }
    frame "PXI-6284" {
    }
    frame "PXI-6289" {
    }
    frame "PXI-6503" {
    }
    frame "PXI-6504" {
    }
    frame "PXI-6505" {
    }
    frame "PXI-6508" {
    }
    frame "PXI-6509" {
    }
    frame "PXI-6511" {
    }
    frame "PXI-6512" {
    }
    frame "PXI-6513" {
    }
    frame "PXI-6514" {
    }
    frame "PXI-6515" {
    }
    frame "PXI-6521" {
    }
    frame "PXI-6525" {
    }
    frame "PXI-6526" {
    }
    frame "PXI-6527" {
    }
    frame "PXI-6528" {
    }
    frame "PXI-6529" {
    }
    frame "PXI-6533" {
    }
    frame "PXI-6534" {
    }
    frame "PXI-6541" {
    }
    frame "PXI-6542" {
    }
    frame "PXI-6551" {
    }
    frame "PXI-6552" {
    }
    frame "PXI-6561" {
    }
    frame "PXI-6562" {
    }
    frame "PXI-6601" {
    }
    frame "PXI-6602" {
    }
    frame "PXI-6608" {
    }
    frame "PXI-6610" {
    }
    frame "PXI-6624" {
    }
    frame "PXI-6651" {
    }
    frame "PXI-6652" {
    }
    frame "PXI-6653" {
    }
    frame "PXI-6682" {
    }
    frame "PXI-6682H" {
    }
    frame "PXI-6683" {
    }
    frame "PXI-6683H" {
    }
    frame "PXI-6684" {
    }
    frame "PXI-6684H" {
    }
    frame "PXI-6685" {
    }
    frame "PXI-6685H" {
    }
    frame "PXI-6703" {
    }
    frame "PXI-6704" {
    }
    frame "PXI-6711" {
    }
    frame "PXI-6713" {
    }
    frame "PXI-6722" {
    }
    frame "PXI-6723" {
    }
    frame "PXI-6731" {
    }
    frame "PXI-6733" {
    }
    frame "PXI-6810" {
    }
    frame "PXI-6830" {
    }
    frame "PXI-7030/6030E" {
    }
    frame "PXI-7040/6040E" {
    }
    frame "PXI-7041/6040E" {
    }
    frame "PXI-7312" {
    }
    frame "PXI-7314" {
    }
    frame "PXI-7322" {
    }
    frame "PXI-7324" {
    }
    frame "PXI-7330" {
    }
    frame "PXI-7332" {
    }
    frame "PXI-7334" {
    }
    frame "PXI-7340" {
    }
    frame "PXI-7342" {
    }
    frame "PXI-7344" {
    }
    frame "PXI-7346" {
    }
    frame "PXI-7350" {
    }
    frame "PXI-7811R" {
    }
    frame "PXI-7813R" {
    }
    frame "PXI-7830R" {
    }
    frame "PXI-7831R" {
    }
    frame "PXI-7833R" {
    }
    frame "PXI-7841R" {
    }
    frame "PXI-7842R" {
    }
    frame "PXI-7851R" {
    }
    frame "PXI-7852R" {
    }
    frame "PXI-7853R" {
    }
    frame "PXI-7854R" {
    }
    frame "PXI-7951R" {
    }
    frame "PXI-7952R" {
    }
    frame "PXI-7953R" {
    }
    frame "PXI-7954R" {
    }
    frame "PXI-8105" {
    }
    frame "PXI-8106" {
    }
    frame "PXI-8107" {
    }
    frame "PXI-8108" {
    }
    frame "PXI-8110" {
    }
    frame "PXI-8115" {
    }
    frame "PXI-8119" {
    }
    frame "PXI-8156B" {
    }
    frame "PXI-8184" {
    }
    frame "PXI-8195" {
    }
    frame "PXI-8250" {
    }
    frame "PXI-8252" {
    }
    frame "PXI-8320" {
    }
    frame "PXI-8352" {
    }
    frame "PXI-8420/16" {
    }
    frame "PXI-8420/2" {
    }
    frame "PXI-8420/4" {
    }
    frame "PXI-8420/8" {
    }
    frame "PXI-8421/2" {
    }
    frame "PXI-8421/4" {
    }
    frame "PXI-8422/2" {
    }
    frame "PXI-8422/4" {
    }
    frame "PXI-8423/2" {
    }
    frame "PXI-8423/4" {
    }
    frame "PXI-8430/16" {
    }
    frame "PXI-8430/2" {
    }
    frame "PXI-8430/4" {
    }
    frame "PXI-8430/8" {
    }
    frame "PXI-8431/2" {
    }
    frame "PXI-8431/4" {
    }
    frame "PXI-8431/8" {
    }
    frame "PXI-8432/2" {
    }
    frame "PXI-8432/4" {
    }
    frame "PXI-8433/2" {
    }
    frame "PXI-8433/4" {
    }
    frame "PXI-8460/1" {
    }
    frame "PXI-8460/1 Series 2" {
    }
    frame "PXI-8460/2" {
    }
    frame "PXI-8460/2 Series 2" {
    }
    frame "PXI-8461 (DNET)" {
    }
    frame "PXI-8461/1" {
    }
    frame "PXI-8461/1 Series 2" {
    }
    frame "PXI-8461/2" {
    }
    frame "PXI-8461/2 Series 2" {
    }
    frame "PXI-8462" {
    }
    frame "PXI-8462 Series 2" {
    }
    frame "PXI-8463/1 Series 2" {
    }
    frame "PXI-8463/2 Series 2" {
    }
    frame "PXI-8464/1" {
    }
    frame "PXI-8464/2 Series 2" {
    }
    frame "PXI-8533" {
    }
    frame "PXI-GPIB" {
    }
    frame "PXIe-1435" {
    }
    frame "PXIe-2512" {
    }
    frame "PXIe-2514" {
    }
    frame "PXIe-2515" {
    }
    frame "PXIe-2524" {
    }
    frame "PXIe-2525" {
    }
    frame "PXIe-2526" {
    }
    frame "PXIe-2527" {
    }
    frame "PXIe-2529" {
    }
    frame "PXIe-2530" {
    }
    frame "PXIe-2531" {
    }
    frame "PXIe-2532" {
    }
    frame "PXIe-2540" {
    }
    frame "PXIe-2541" {
    }
    frame "PXIe-2542" {
    }
    frame "PXIe-2543" {
    }
    frame "PXIe-2544" {
    }
    frame "PXIe-2569" {
    }
    frame "PXIe-2575" {
    }
    frame "PXIe-2593" {
    }
    frame "PXIe-2725" {
    }
    frame "PXIe-2727" {
    }
    frame "PXIe-2737" {
    }
    frame "PXIe-2738" {
    }
    frame "PXIe-2739" {
    }
    frame "PXIe-2746" {
    }
    frame "PXIe-2747" {
    }
    frame "PXIe-2748" {
    }
    frame "PXIe-2790" {
    }
    frame "PXIe-3610" {
    }
    frame "PXIe-3620" {
    }
    frame "PXIe-3630" {
    }
    frame "PXIe-3647" {
    }
    frame "PXIe-3657" {
    }
    frame "PXIe-4080" {
    }
    frame "PXIe-4081" {
    }
    frame "PXIe-4082" {
    }
    frame "PXIe-4135" {
    }
    frame "PXIe-4300" {
    }
    frame "PXIe-4302" {
    }
    frame "PXIe-4303" {
    }
    frame "PXIe-4304" {
    }
    frame "PXIe-4305" {
    }
    frame "PXIe-4309" {
    }
    frame "PXIe-4310" {
    }
    frame "PXIe-4322" {
    }
    frame "PXIe-4330" {
    }
    frame "PXIe-4331" {
    }
    frame "PXIe-4339" {
    }
    frame "PXIe-4340" {
    }
    frame "PXIe-4353" {
    }
    frame "PXIe-4357" {
    }
    frame "PXIe-4463" {
    }
    frame "PXIe-4464" {
    }
    frame "PXIe-4480" {
    }
    frame "PXIe-4481" {
    }
    frame "PXIe-4492" {
    }
    frame "PXIe-4497" {
    }
    frame "PXIe-4499" {
    }
    frame "PXIe-4844 (OSI)" {
    }
    frame "PXIe-5105" {
    }
    frame "PXIe-5114" {
    }
    frame "PXIe-5160 (2 ch)" {
    }
    frame "PXIe-5160 (4 ch)" {
    }
    frame "PXIe-5162 (2 ch)" {
    }
    frame "PXIe-5162 (4 ch)" {
    }
    frame "PXIe-5164" {
    }
    frame "PXIe-5170R" {
    }
    frame "PXIe-5171R" {
    }
    frame "PXIe-5172" {
    }
    frame "PXIe-5185 (1 MOhm)" {
    }
    frame "PXIe-5185 (50 Ohm)" {
    }
    frame "PXIe-5186 (1 MOhm)" {
    }
    frame "PXIe-5186 (50 Ohm)" {
    }
    frame "PXIe-5601" {
    }
    frame "PXIe-5603" {
    }
    frame "PXIe-5605" {
    }
    frame "PXIe-5606" {
    }
    frame "PXIe-5611" {
    }
    frame "PXIe-5624" {
    }
    frame "PXIe-5630" {
    }
    frame "PXIe-5632" {
    }
    frame "PXIe-5641R" {
    }
    frame "PXIe-5644R" {
    }
    frame "PXIe-5645R" {
    }
    frame "PXIe-5646R" {
    }
    frame "PXIe-5650" {
    }
    frame "PXIe-5651" {
    }
    frame "PXIe-5652" {
    }
    frame "PXIe-5653" {
    }
    frame "PXIe-5654" {
    }
    frame "PXIe-5663" {
    }
    frame "PXIe-5663E" {
    }
    frame "PXIe-5665 14GHz" {
    }
    frame "PXIe-5665 3.6GHz" {
    }
    frame "PXIe-5667 3.6GHz" {
    }
    frame "PXIe-5667 7GHz" {
    }
    frame "PXIe-5668R" {
    }
    frame "PXIe-5672" {
    }
    frame "PXIe-5673" {
    }
    frame "PXIe-5693" {
    }
    frame "PXIe-5694" {
    }
    frame "PXIe-5698" {
    }
    frame "PXIe-5840" {
    }
    frame "PXIe-6124" {
    }
    frame "PXIe-6341" {
    }
    frame "PXIe-6346" {
    }
    frame "PXIe-6356" {
    }
    frame "PXIe-6358" {
    }
    frame "PXIe-6361" {
    }
    frame "PXIe-6363" {
    }
    frame "PXIe-6366" {
    }
    frame "PXIe-6368" {
    }
    frame "PXIe-6376" {
    }
    frame "PXIe-6378" {
    }
    frame "PXIe-6544" {
    }
    frame "PXIe-6545" {
    }
    frame "PXIe-6547" {
    }
    frame "PXIe-6548" {
    }
    frame "PXIe-6555" {
    }
    frame "PXIe-6556" {
    }
    frame "PXIe-6570" {
    }
    frame "PXIe-6612" {
    }
    frame "PXIe-6614" {
    }
    frame "PXIe-6672" {
    }
    frame "PXIe-6674" {
    }
    frame "PXIe-6674T" {
    }
    frame "PXIe-6738" {
    }
    frame "PXIe-6739" {
    }
    frame "PXIe-7820R" {
    }
    frame "PXIe-7821R" {
    }
    frame "PXIe-7822R" {
    }
    frame "PXIe-7846R" {
    }
    frame "PXIe-7847R" {
    }
    frame "PXIe-7856R" {
    }
    frame "PXIe-7857R" {
    }
    frame "PXIe-7858R" {
    }
    frame "PXIe-7961R" {
    }
    frame "PXIe-7962R" {
    }
    frame "PXIe-7965R" {
    }
    frame "PXIe-7966R" {
    }
    frame "PXIe-7971R" {
    }
    frame "PXIe-7972R" {
    }
    frame "PXIe-7975R" {
    }
    frame "PXIe-7976R" {
    }
    frame "PXIe-8100" {
    }
    frame "PXIe-8115" {
    }
    frame "PXIe-8135" {
    }
    frame "PXIe-8364 (NT)" {
    }
    frame "PXIe-8374 (NT)" {
    }
    frame "PXIe-8378" {
    }
    frame "PXIe-8379" {
    }
    frame "PXIe-8383mc" {
    }
    frame "PXIe-8384" {
    }
    frame "PXIe-8388" {
    }
    frame "PXIe-8389" {
    }
    frame "PXIe-8510" {
    }
    frame "SB-A2200" {
    }
    frame "SB-MIO-16E-4" {
    }
    frame "SC-2040" {
    }
    frame "SC-2042-RTD" {
    }
    frame "SC-2043-SG" {
    }
    frame "SC-2050" {
    }
    frame "SC-2051" {
    }
    frame "SC-2052" {
    }
    frame "SC-2053" {
    }
    frame "SC-2054" {
    }
    frame "SC-2055" {
    }
    frame "SC-2056" {
    }
    frame "SC-2060" {
    }
    frame "SC-2061" {
    }
    frame "SC-2062" {
    }
    frame "SC-2070" {
    }
    frame "SC-2071" {
    }
    frame "SC-2072" {
    }
    frame "SC-2072D" {
    }
    frame "SC-2075" {
    }
    frame "SC-2311" {
    }
    frame "SC-2345" {
    }
    frame "SC-2350" {
    }
    frame "SCB-100" {
    }
    frame "SCB-68" {
    }
    frame "SCB-68A" {
    }
    frame "SCC-68" {
    }
    frame "SCC-A10" {
    }
    frame "SCC-AI00" {
    }
    frame "SCC-AI01" {
    }
    frame "SCC-AI02" {
    }
    frame "SCC-AI03" {
    }
    frame "SCC-AI04" {
    }
    frame "SCC-AI05" {
    }
    frame "SCC-AI06" {
    }
    frame "SCC-AI07" {
    }
    frame "SCC-AI13" {
    }
    frame "SCC-AI14" {
    }
    frame "SCC-AI16" {
    }
    frame "SCC-AO10" {
    }
    frame "SCC-CI20" {
    }
    frame "SCC-CO20" {
    }
    frame "SCC-CTR01" {
    }
    frame "SCC-DI01" {
    }
    frame "SCC-DO01" {
    }
    frame "SCC-FT01" {
    }
    frame "SCC-FV01" {
    }
    frame "SCC-LP01" {
    }
    frame "SCC-LP02" {
    }
    frame "SCC-LP03" {
    }
    frame "SCC-LP04" {
    }
    frame "SCC-LP05" {
    }
    frame "SCC-PWR01" {
    }
    frame "SCC-PWR02" {
    }
    frame "SCC-PWR03" {
    }
    frame "SCC-RLY01" {
    }
    frame "SCC-RTD01" {
    }
    frame "SCC-SG01" {
    }
    frame "SCC-SG02" {
    }
    frame "SCC-SG03" {
    }
    frame "SCC-SG04" {
    }
    frame "SCC-SG11" {
    }
    frame "SCC-SG24" {
    }
    frame "SCC-TC01" {
    }
    frame "SCC-TC02" {
    }
    frame "SCC-TC03" {
    }
    frame "SCC-TC12" {
    }
    frame "SCC-TC13" {
    }
    frame "SCMP-100uA" {
    }
    frame "SCMP-10V" {
    }
    frame "SCMP-10uA" {
    }
    frame "SCMP-13mA" {
    }
    frame "SCMP-1V" {
    }
    frame "SCMP-1mA" {
    }
    frame "SCMP-2V" {
    }
    frame "SCMP-5V" {
    }
    frame "SCXI-1000" {
    }
    frame "SCXI-1000DC" {
    }
    frame "SCXI-1001" {
    }
    frame "SCXI-1100" {
    }
    frame "SCXI-1101" {
    }
    frame "SCXI-1102" {
    }
    frame "SCXI-1102B" {
    }
    frame "SCXI-1102C" {
    }
    frame "SCXI-1104" {
    }
    frame "SCXI-1104C" {
    }
    frame "SCXI-1112" {
    }
    frame "SCXI-1120" {
    }
    frame "SCXI-1120D" {
    }
    frame "SCXI-1121" {
    }
    frame "SCXI-1122" {
    }
    frame "SCXI-1124" {
    }
    frame "SCXI-1125" {
    }
    frame "SCXI-1126" {
    }
    frame "SCXI-1127" {
    }
    frame "SCXI-1128" {
    }
    frame "SCXI-1129" {
    }
    frame "SCXI-1130" {
    }
    frame "SCXI-1140" {
    }
    frame "SCXI-1141" {
    }
    frame "SCXI-1142" {
    }
    frame "SCXI-1143" {
    }
    frame "SCXI-1160" {
    }
    frame "SCXI-1160A" {
    }
    frame "SCXI-1161" {
    }
    frame "SCXI-1162" {
    }
    frame "SCXI-1162HV" {
    }
    frame "SCXI-1163" {
    }
    frame "SCXI-1163R" {
    }
    frame "SCXI-1166" {
    }
    frame "SCXI-1167" {
    }
    frame "SCXI-1169" {
    }
    frame "SCXI-1175" {
    }
    frame "SCXI-1190" {
    }
    frame "SCXI-1191" {
    }
    frame "SCXI-1192" {
    }
    frame "SCXI-1193" {
    }
    frame "SCXI-1194" {
    }
    frame "SCXI-1195" {
    }
    frame "SCXI-1200" {
    }
    frame "SCXI-1300" {
    }
    frame "SCXI-1301" {
    }
    frame "SCXI-1302" {
    }
    frame "SCXI-1303" {
    }
    frame "SCXI-1304" {
    }
    frame "SCXI-1305" {
    }
    frame "SCXI-1306" {
    }
    frame "SCXI-1307" {
    }
    frame "SCXI-1308" {
    }
    frame "SCXI-1310" {
    }
    frame "SCXI-1311" {
    }
    frame "SCXI-1313" {
    }
    frame "SCXI-1314" {
    }
    frame "SCXI-1314T" {
    }
    frame "SCXI-1315" {
    }
    frame "SCXI-1317" {
    }
    frame "SCXI-1320" {
    }
    frame "SCXI-1321" {
    }
    frame "SCXI-1322" {
    }
    frame "SCXI-1323" {
    }
    frame "SCXI-1324" {
    }
    frame "SCXI-1325" {
    }
    frame "SCXI-1326" {
    }
    frame "SCXI-1327" {
    }
    frame "SCXI-1328" {
    }
    frame "SCXI-1330" {
    }
    frame "SCXI-1331" {
    }
    frame "SCXI-1332" {
    }
    frame "SCXI-1333" {
    }
    frame "SCXI-1334" {
    }
    frame "SCXI-1335" {
    }
    frame "SCXI-1336" {
    }
    frame "SCXI-1337" {
    }
    frame "SCXI-1338" {
    }
    frame "SCXI-1339" {
    }
    frame "SCXI-1357" {
    }
    frame "SCXI-1366" {
    }
    frame "SCXI-1377" {
    }
    frame "SCXI-1378" {
    }
    frame "SCXI-1379" {
    }
    frame "SCXI-1502" {
    }
    frame "SCXI-1503" {
    }
    frame "SCXI-1520" {
    }
    frame "SCXI-1521" {
    }
    frame "SCXI-1521B" {
    }
    frame "SCXI-1530" {
    }
    frame "SCXI-1531" {
    }
    frame "SCXI-1540" {
    }
    frame "SCXI-1581" {
    }
    frame "SCXI-1600" {
    }
    frame "SCXI-2000" {
    }
    frame "SCXI-2400" {
    }
    frame "SSR-BP16" {
    }
    frame "SSR-BP24" {
    }
    frame "SSR-BP32" {
    }
    frame "SSR-BP8" {
    }
    frame "SSR-IAC-5" {
    }
    frame "SSR-IAC-5A" {
    }
    frame "SSR-IDC-5" {
    }
    frame "SSR-OAC-5" {
    }
    frame "SSR-OAC-5A" {
    }
    frame "SSR-ODC-5" {
    }
    frame "SensorDAQ" {
    }
    frame "TB-2130" {
    }
    frame "TB-2605" {
    }
    frame "TB-2606" {
    }
    frame "TB-2621" {
    }
    frame "TB-2627" {
    }
    frame "TB-2630" {
    }
    frame "TB-2630B" {
    }
    frame "TB-2631" {
    }
    frame "TB-2632" {
    }
    frame "TB-2634" {
    }
    frame "TB-2635" {
    }
    frame "TB-2636" {
    }
    frame "TB-2640" {
    }
    frame "TB-2641" {
    }
    frame "TB-2642" {
    }
    frame "TB-2643" {
    }
    frame "TB-2644" {
    }
    frame "TB-2645" {
    }
    frame "TB-2646" {
    }
    frame "TB-2666" {
    }
    frame "TB-2676" {
    }
    frame "TB-2705" {
    }
    frame "TB-2706" {
    }
    frame "TB-2708" {
    }
    frame "TB-2709" {
    }
    frame "TB-2715" {
    }
    frame "TB-2725" {
    }
    frame "TB-4300C" {
    }
    frame "TB-4302" {
    }
    frame "TB-4302C" {
    }
    frame "TB-4304" {
    }
    frame "TB-4339" {
    }
    frame "TB-4339B" {
    }
    frame "TB-4339C" {
    }
    frame "TB-4357" {
    }
    frame "TBX-1303" {
    }
    frame "TBX-1316" {
    }
    frame "TBX-1325" {
    }
    frame "TBX-1326" {
    }
    frame "TBX-1328" {
    }
    frame "TBX-1329" {
    }
    frame "TBX-2131" {
    }
    frame "TBX-24F" {
    }
    frame "TBX-68" {
    }
    frame "TBX-68T" {
    }
    frame "TBX-96" {
    }
    frame "TC-2095" {
    }
    frame "TC-2190" {
    }
    frame "TC-4353" {
    }
    frame "USB-1359" {
    }
    frame "USB-232" {
    }
    frame "USB-232/2" {
    }
    frame "USB-232/4" {
    }
    frame "USB-4065" {
    }
    frame "USB-4431" {
    }
    frame "USB-4432" {
    }
    frame "USB-4444" {
    }
    frame "USB-485" {
    }
    frame "USB-485/2" {
    }
    frame "USB-485/4" {
    }
    frame "USB-488" {
    }
    frame "USB-5132" {
    }
    frame "USB-5133" {
    }
    frame "USB-5134" {
    }
    frame "USB-5680" {
    }
    frame "USB-5681" {
    }
    frame "USB-5683" {
    }
    frame "USB-5684" {
    }
    frame "USB-6000" {
    }
    frame "USB-6000 OEM" {
    }
    frame "USB-6002" {
    }
    frame "USB-6002 OEM" {
    }
    frame "USB-6003" {
    }
    frame "USB-6003 OEM" {
    }
    frame "USB-6005" {
    }
    frame "USB-6005 OEM" {
    }
    frame "USB-6005 VSA" {
    }
    frame "USB-6008" {
    }
    frame "USB-6009" {
    }
    frame "USB-6009 OEM" {
    }
    frame "USB-6210" {
    }
    frame "USB-6210 OEM" {
    }
    frame "USB-6211" {
    }
    frame "USB-6211 OEM" {
    }
    frame "USB-6212" {
    }
    frame "USB-6212 BNC" {
    }
    frame "USB-6212 Mass Term" {
    }
    frame "USB-6212 OEM" {
    }
    frame "USB-6215" {
    }
    frame "USB-6215 OEM" {
    }
    frame "USB-6216" {
    }
    frame "USB-6216 BNC" {
    }
    frame "USB-6216 Mass Term" {
    }
    frame "USB-6216 OEM" {
    }
    frame "USB-6218" {
    }
    frame "USB-6218 BNC" {
    }
    frame "USB-6218 OEM" {
    }
    frame "USB-6220" {
    }
    frame "USB-6220 Mass Term" {
    }
    frame "USB-6220 OEM" {
    }
    frame "USB-6221" {
    }
    frame "USB-6221 (BNC)" {
    }
    frame "USB-6221 BNC" {
    }
    frame "USB-6221 Mass Term" {
    }
    frame "USB-6221 OEM" {
    }
    frame "USB-6224" {
    }
    frame "USB-6224 Mass Term" {
    }
    frame "USB-6224 OEM" {
    }
    frame "USB-6225" {
    }
    frame "USB-6225 Mass Term" {
    }
    frame "USB-6229" {
    }
    frame "USB-6229 (BNC)" {
    }
    frame "USB-6229 BNC" {
    }
    frame "USB-6229 Mass Term" {
    }
    frame "USB-6229 OEM" {
    }
    frame "USB-6250" {
    }
    frame "USB-6250 Mass Term" {
    }
    frame "USB-6250 OEM" {
    }
    frame "USB-6251" {
    }
    frame "USB-6251 (BNC)" {
    }
    frame "USB-6251 BNC" {
    }
    frame "USB-6251 Mass Term" {
    }
    frame "USB-6251 OEM" {
    }
    frame "USB-6254" {
    }
    frame "USB-6254 Mass Term" {
    }
    frame "USB-6254 OEM" {
    }
    frame "USB-6255" {
    }
    frame "USB-6255 Mass Term" {
    }
    frame "USB-6259" {
    }
    frame "USB-6259 (BNC)" {
    }
    frame "USB-6259 BNC" {
    }
    frame "USB-6259 Mass Term" {
    }
    frame "USB-6259 OEM" {
    }
    frame "USB-6281" {
    }
    frame "USB-6281 (Mass Termination)" {
    }
    frame "USB-6281 BNC" {
    }
    frame "USB-6281 Mass Term" {
    }
    frame "USB-6289" {
    }
    frame "USB-6289 (Mass Termination)" {
    }
    frame "USB-6289 BNC" {
    }
    frame "USB-6289 Mass Term" {
    }
    frame "USB-6326" {
    }
    frame "USB-6341 BNC" {
    }
    frame "USB-6343 BNC" {
    }
    frame "USB-6343 OEM RTSI" {
    }
    frame "USB-6346" {
    }
    frame "USB-6356 (32MS) BNC" {
    }
    frame "USB-6356 (32MS) OEM RTSI" {
    }
    frame "USB-6361 BNC" {
    }
    frame "USB-6363 BNC" {
    }
    frame "USB-6363 Mass Term RTSI" {
    }
    frame "USB-6366 (64MS) BNC" {
    }
    frame "USB-6501" {
    }
    frame "USB-6504" {
    }
    frame "USB-6509" {
    }
    frame "USB-6525" {
    }
    frame "USB-7931R" {
    }
    frame "USB-7932R" {
    }
    frame "USB-7933R" {
    }
    frame "USB-8451" {
    }
    frame "USB-8452" {
    }
    frame "USB-8472" {
    }
    frame "USB-8472s" {
    }
    frame "USB-8473" {
    }
    frame "USB-8473s" {
    }
    frame "USB-8476" {
    }
    frame "USB-8476s" {
    }
    frame "USB-8502" {
    }
    frame "USB-8506" {
    }
    frame "USB-9161" {
    }
    frame "USB-9162" {
    }
    frame "USB-9201" {
    }
    frame "USB-9201 D-Sub" {
    }
    frame "USB-9211" {
    }
    frame "USB-9211A" {
    }
    frame "USB-9213" {
    }
    frame "USB-9215" {
    }
    frame "USB-9215A" {
    }
    frame "USB-9215A BNC" {
    }
    frame "USB-9221" {
    }
    frame "USB-9229 (BNC)" {
    }
    frame "USB-9233" {
    }
    frame "USB-9234" {
    }
    frame "USB-9237" {
    }
    frame "USB-9239 (BNC)" {
    }
    frame "USB-9263 (BNC)" {
    }
    frame "USB-9264 D-SUB" {
    }
    frame "USB-9421" {
    }
    frame "USB-9421 D-Sub" {
    }
    frame "USB-9421DSUB" {
    }
    frame "USB-9472" {
    }
    frame "USB-9472 D-Sub" {
    }
    frame "USB-9472DSUB" {
    }
    frame "USB-9481" {
    }
    frame "VMEpc-650" {
    }
    frame "VXI-1394" {
    }
    frame "VXI-2701" {
    }
    frame "VXI-2703" {
    }
    frame "VXI-2727" {
    }
    frame "VXI-5412" {
    }
    frame "VXI-5432" {
    }
    frame "VXI-5912" {
    }
    frame "VXI-8340" {
    }
    frame "VXI-8345" {
    }
    frame "VXI-AO-48XDC" {
    }
    frame "VXI-DIO-128" {
    }
    frame "VXI-MIO-64E-1" {
    }
    frame "VXI-MIO-64XE-10" {
    }
    frame "VXI-SC-1000" {
    }
    frame "VXI-SC-1102" {
    }
    frame "VXI-SC-1102B" {
    }
    frame "VXI-SC-1102C" {
    }
    frame "VXI-SC-1150" {
    }
    frame "VXI-TB-1303" {
    }
    frame "VXI-TB-96" {
    }
    frame "VXI-USB" {
    }
    frame "VXIpc-650" {
    }
    frame "VXIpc-740" {
    }
    frame "VXIpc-770" {
    }
    frame "VXIpc-850" {
    }
    frame "VXIpc-860" {
    }
    frame "VXIpc-870" {
    }
    frame "VXIpc-870B" {
    }
    frame "VXIpc-881" {
    }
    frame "WLAN Toolkit" {
    }
    frame "WLS-9205" {
    }
    frame "WLS-9205 DSUB" {
    }
    frame "WLS-9206" {
    }
    frame "WLS-9211" {
    }
    frame "WLS-9213" {
    }
    frame "WLS-9215" {
    }
    frame "WLS-9215 BNC" {
    }
    frame "WLS-9219" {
    }
    frame "WLS-9234" {
    }
    frame "WLS-9237" {
    }
    frame "WLS-9421" {
    }
    frame "WLS-9421 DSUB" {
    }
    frame "WLS-9472" {
    }
    frame "WLS-9472 DSUB" {
    }
    frame "WLS-9481" {
    }
    frame "cDAQ-9171" {
    }
    frame "cDAQ-9171 OEM" {
    }
    frame "cDAQ-9172" {
    }
    frame "cDAQ-9174" {
    }
    frame "cDAQ-9178" {
    }
    frame "cDAQ-9181" {
    }
    frame "cDAQ-9184" {
    }
    frame "cDAQ-9188" {
    }
    frame "cDAQ-9191" {
    }
    frame "cFP-1804" {
    }
    frame "cFP-1808" {
    }
    frame "cFP-2000" {
    }
    frame "cFP-2010" {
    }
    frame "cFP-2020" {
    }
    frame "cFP-2100" {
    }
    frame "cFP-2110" {
    }
    frame "cFP-2120" {
    }
    frame "cFP-2200" {
    }
    frame "cFP-AI-100" {
    }
    frame "cFP-AI-102" {
    }
    frame "cFP-AI-110" {
    }
    frame "cFP-AI-111" {
    }
    frame "cFP-AI-112" {
    }
    frame "cFP-AI-118" {
    }
    frame "cFP-AIO-600" {
    }
    frame "cFP-AIO-610" {
    }
    frame "cFP-AO-200" {
    }
    frame "cFP-AO-210" {
    }
    frame "cFP-CTR-500" {
    }
    frame "cFP-CTR-502" {
    }
    frame "cFP-DI-300" {
    }
    frame "cFP-DI-301" {
    }
    frame "cFP-DI-304" {
    }
    frame "cFP-DI-330" {
    }
    frame "cFP-DIO-550" {
    }
    frame "cFP-DO-400" {
    }
    frame "cFP-DO-401" {
    }
    frame "cFP-DO-403" {
    }
    frame "cFP-DO-404" {
    }
    frame "cFP-DO-410" {
    }
    frame "cFP-PG-522" {
    }
    frame "cFP-PWM-520" {
    }
    frame "cFP-QUAD-510" {
    }
    frame "cFP-RLY-420" {
    }
    frame "cFP-RLY-421" {
    }
    frame "cFP-RLY-422" {
    }
    frame "cFP-RLY-423" {
    }
    frame "cFP-RLY-425" {
    }
    frame "cFP-RTD-122" {
    }
    frame "cFP-RTD-124" {
    }
    frame "cFP-SG-140" {
    }
    frame "cFP-TC-120" {
    }
    frame "cFP-TC-125" {
    }
    frame "cRIO-9002" {
    }
    frame "cRIO-9004" {
    }
    frame "cRIO-9012" {
    }
    frame "cRIO-9014" {
    }
    frame "cRIO-9022" {
    }
    frame "cRIO-9023" {
    }
    frame "cRIO-9024" {
    }
    frame "cRIO-9025" {
    }
    frame "cRIO-9030" {
    }
    frame "cRIO-9031" {
    }
    frame "cRIO-9032" {
    }
    frame "cRIO-9033" {
    }
    frame "cRIO-9034" {
    }
    frame "cRIO-9035" {
    }
    frame "cRIO-9036" {
    }
    frame "cRIO-9037" {
    }
    frame "cRIO-9038" {
    }
    frame "cRIO-9039" {
    }
    frame "cRIO-9063" {
    }
    frame "cRIO-9064" {
    }
    frame "cRIO-9065" {
    }
    frame "cRIO-9066" {
    }
    frame "cRIO-9067" {
    }
    frame "cRIO-9068" {
    }
    frame "cRIO-9072" {
    }
    frame "cRIO-9073" {
    }
    frame "cRIO-9074" {
    }
    frame "cRIO-9075" {
    }
    frame "cRIO-9076" {
    }
    frame "cRIO-9077" {
    }
    frame "cRIO-9081" {
    }
    frame "cRIO-9082" {
    }
    frame "cRIO-9101" {
    }
    frame "cRIO-9102" {
    }
    frame "cRIO-9103" {
    }
    frame "cRIO-9104" {
    }
    frame "cRIO-9111" {
    }
    frame "cRIO-9112" {
    }
    frame "cRIO-9113" {
    }
    frame "cRIO-9114" {
    }
    frame "cRIO-9116" {
    }
    frame "cRIO-9118" {
    }
    frame "cRIO-9413" {
    }
    frame "cRIO-FRC II" {
    }
    frame "sbRIO-9601" {
    }
    frame "sbRIO-9602" {
    }
    frame "sbRIO-9603" {
    }
    frame "sbRIO-9605" {
    }
    frame "sbRIO-9606" {
    }
    frame "sbRIO-9607" {
    }
    frame "sbRIO-9611" {
    }
    frame "sbRIO-9612" {
    }
    frame "sbRIO-9623" {
    }
    frame "sbRIO-9625" {
    }
    frame "sbRIO-9626" {
    }
    frame "sbRIO-9627" {
    }
    frame "sbRIO-9631" {
    }
    frame "sbRIO-9632" {
    }
    frame "sbRIO-9633" {
    }
    frame "sbRIO-9636" {
    }
    frame "sbRIO-9637" {
    }
    frame "sbRIO-9641" {
    }
    frame "sbRIO-9642" {
    }
    frame "sbRIO-9651" {
    }
  }
